vi "rio_veloster12.vi"() -> ()   [LabVIEW 2015]
uses:
  <vilib>/FPGAPlugInAG/cRIO-9113/niLvFpga_Open_cRIO-9113.vi
  <vilib>/rvi/interface/common/dynamic/niFpgaDynamicAddResources.vi
  <vilib>/FPGAPlugInAG/Dynamic/niLvFpga_Abort_Dynamic.vi
  <vilib>/FPGAPlugInAG/Dynamic/niLvFpga_Run_Dynamic.vi
  rio_Global.vi
  <vilib>/Utility/error.llb/Error Cluster From Error Code.vi
  <vilib>/rvi/errors/niLvFpgaAdjustHostInterfaceError.vi
  <vilib>/Instr/_visa.llb/VISA Configure Serial Port (Instr).vi
  <vilib>/Analysis/Matrix/Numeric/Conversions/Array To Matrix - RA2.vi
  <vilib>/Analysis/Matrix/Numeric/Multiply/Multiply - RM,RM.vi
  <vilib>/Analysis/Matrix/Numeric/Add/Add - RM,RM.vi
  <vilib>/Analysis/baseanly.llb/Real Inverse Matrix.vi
  <vilib>/Analysis/Matrix/Numeric/Subtract/Subtract - RM,RM.vi
  <vilib>/Analysis/Matrix/Numeric/Conversions/Array To Matrix - RA.vi
  <vilib>/Analysis/Matrix/Numeric/Multiply/Multiply - R,RM.vi
  <vilib>/Analysis/Matrix/Numeric/Conversions/Matrix To Array - RM.vi
  <vilib>/rvi/interface/nirviOpenFPGA/nirviOpenFPGA.xnode
  FPGA Bitfiles/autonomous_FPGATarget2_fpga4_FZHAM7r+pqE.lvbitx
  fpga/fpga4.vi
  <vilib>/rvi/interface/nirviMethod/nirviMethod.xnode
  <vilib>/rvi/interface/nirviReadWriteControl/nirviReadWriteControl.xnode
  <vilib>/Analysis/Matrix/NI_Matrix.lvlib
  <vilib>/Analysis/NI_AALBase.lvlib
  NiFpgaLv.dll
  <vilib>/rvi/interface/Simulation/niFpgaSimulationCallBeginRW.vi
panel:
  out "C_yaw_rate":dbl
  out "Time old":u32[](array[numeric])
  out "Heading":dbl
  out "H_GPS":dbl
  out "pos":dbl[](array[numeric])
  in  "GPS init":bool=TRUE
  out "pos_gps":dbl[](array[numeric]) format="%#_19f"
  out "dt":dbl
  out "Pos_time 10":i32
  out "FPGA":refnum<k20>
  in  "steer limit":dbl=100.0
  in  "buzz":bool
  out "hcount":u64=1
  out "hbias":dbl
  out "vcount":u64=1
  out "vgain":dbl=1.0
  out "T PWM":u16
  out "B PWM":u16
  out "mobileye":u8[](array[numeric])
  out "timer":u32
  out "Mobileye_time 100":u32
  out "pos error":dbl
  in  "Gear Manual":i32(slide)=1 scale=-1.0..1.0
  out "map":i32=2
  out "P, R, D":i32
  out "heading error":dbl
  out "POS init":bool
  out "VS_CAN":dbl
  in  "brake":bool
  in  "Slide":dbl(slide) min=-50.0 max=50.0 step=50.0 scale=-50.0..50.0
  out "Con_time 10":i32
  out "CAN_time 10":u32
  out "ecef ref":dbl[](array[numeric])
  out "h_gps":dbl
  out "get heading":bool
  out "get position":bool
  out "rt":dbl
  out "CAN Comm Enabled":bool
  in  "SPAS Enable":bool=TRUE
  in  "file write":bool
  out "data write":refnum<file>
  out "file rw error":errorcluster
  in  "Steer input":bool=TRUE
  in  "Manual Steering angle":dbl(knob) scale=-550.0..550.0
  out "Ref vel":dbl=1.0
  in  "Manual Speed":dbl
  in  "Velocity input":bool
  out "Auto":bool
  out "Run":bool
  out "E - STOP":bool
  # "P"
  # "R"
  # "D"
  # "Manual Steering angle"
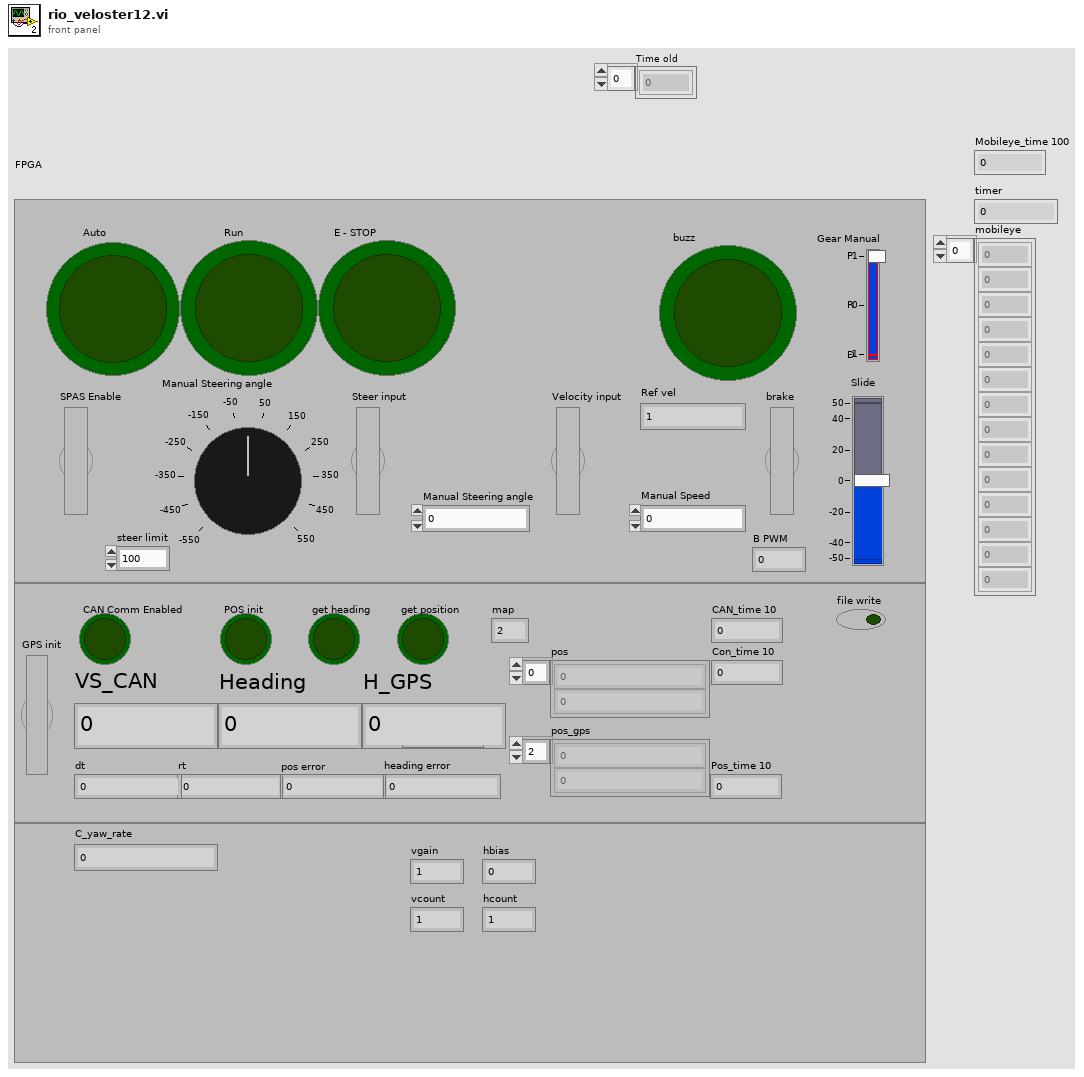
[diagram p1: front panel]
types:
  T1 = enum16{"open", "replace", "create", "open or create", "replace or create", "replace or create with confirmation"}
  T2 = cluster{"timestamp high":u32, "timestamp low":u32, "identifier":u32, "type":enum8{"Data Frame", "Remote Frame", "(reserved)", "(reserved) ", "(reserved)  ", "(reserved)   ", "Bus Error", "Transceiver Fault"}, "info A":u8, "info B":u8, "data length":u8, "data":u8[]}
  T3 = cluster{"identifier":u32, "timestamp":timestamp, "payload":u8[]}
  T4 = cluster{"connection ID":refnum<k16>, "net address":u32, "port":u16}
  T5 = cluster{"hash":i64, "sys time":i64, "mobileye":u8[]}
  T6 = cluster{"hash":i64, "sys time":i64, "time":dbl, "yaw_rate":dbl, "mdps torque":dbl, "mdps str_ang":dbl, "VS_CAN":dbl, "lat_accel":dbl, "mcp":dbl, "accel pedal value":dbl, "tps":dbl, "odometer":dbl, "battery voltage":dbl, "WHL_SPD_RR":dbl, "WHL_SPD_RL":dbl, "WHL_SPD_FR":dbl, "WHL_SPD_FL":dbl}
  T7 = cluster{"hash":i64, "sys time":i64, "ref_vel":dbl, "ref_steer":dbl, "alert":u8}
  T8 = cluster{"hash":i64, "sys time":i64, "ref_vel":dbl, "ref_steer":dbl}
  T9 = cluster{"hash":i64, "sys time":i64, "Auto":bool, "Run":bool, "Solenoid":bool, "T lim":bool, "brk_enc":u8, "B PWM":u16, "T PWM":u16, "ref_vel":dbl, "ref_bkr_enc":dbl, "ref_apv":dbl, "ref_steer":dbl}
  T10 = cluster{"hash":i64, "sys time":i64, "time":dbl, "x":dbl, "y":dbl, "h":dbl, "numSV":i32, "postype":i32, "lag":i32, "hordev":dbl, "lat":dbl, "lon":dbl, "hgt":dbl, "map_idx":i32}
  T11 = cluster{"output[0]":dbl, "output[1]":dbl, "output[2]":dbl, "output[3]":dbl, "output[4]":dbl, "output[5]":dbl, "output[6]":dbl, "output[7]":dbl, "output[8]":dbl, "output[9]":dbl, "output[10]":dbl, "output[11]":dbl, "output[12]":dbl, "output[13]":dbl, "output[14]":dbl}
  T12 = cluster{"hash":i64, "sys time":i64, "time":dbl, "speed":dbl, "heading":dbl, "lat":dbl, "lon":dbl}
  T13 = cluster{"output[0]":dbl, "output[1]":dbl, "output[2]":dbl, "output[3]":dbl, "output[4]":dbl, "output[5]":dbl, "output[6]":dbl}
  T14 = typedef "NI_Matrix.lvlib/RealMatrix.ctl" = dbl[][]
  T15 = cluster{"hash":i64, "sys time":i64, "dt":dbl, "x":dbl, "y":dbl, "speed":dbl, "heading":dbl, "yaw_rate":dbl}
  T16 = cluster{"Real 2D Array[0]":dbl, "Real 2D Array[1]":dbl, "Real 2D Array[2]":dbl, "Real 2D Array[3]":dbl, "Real 2D Array[4]":dbl}
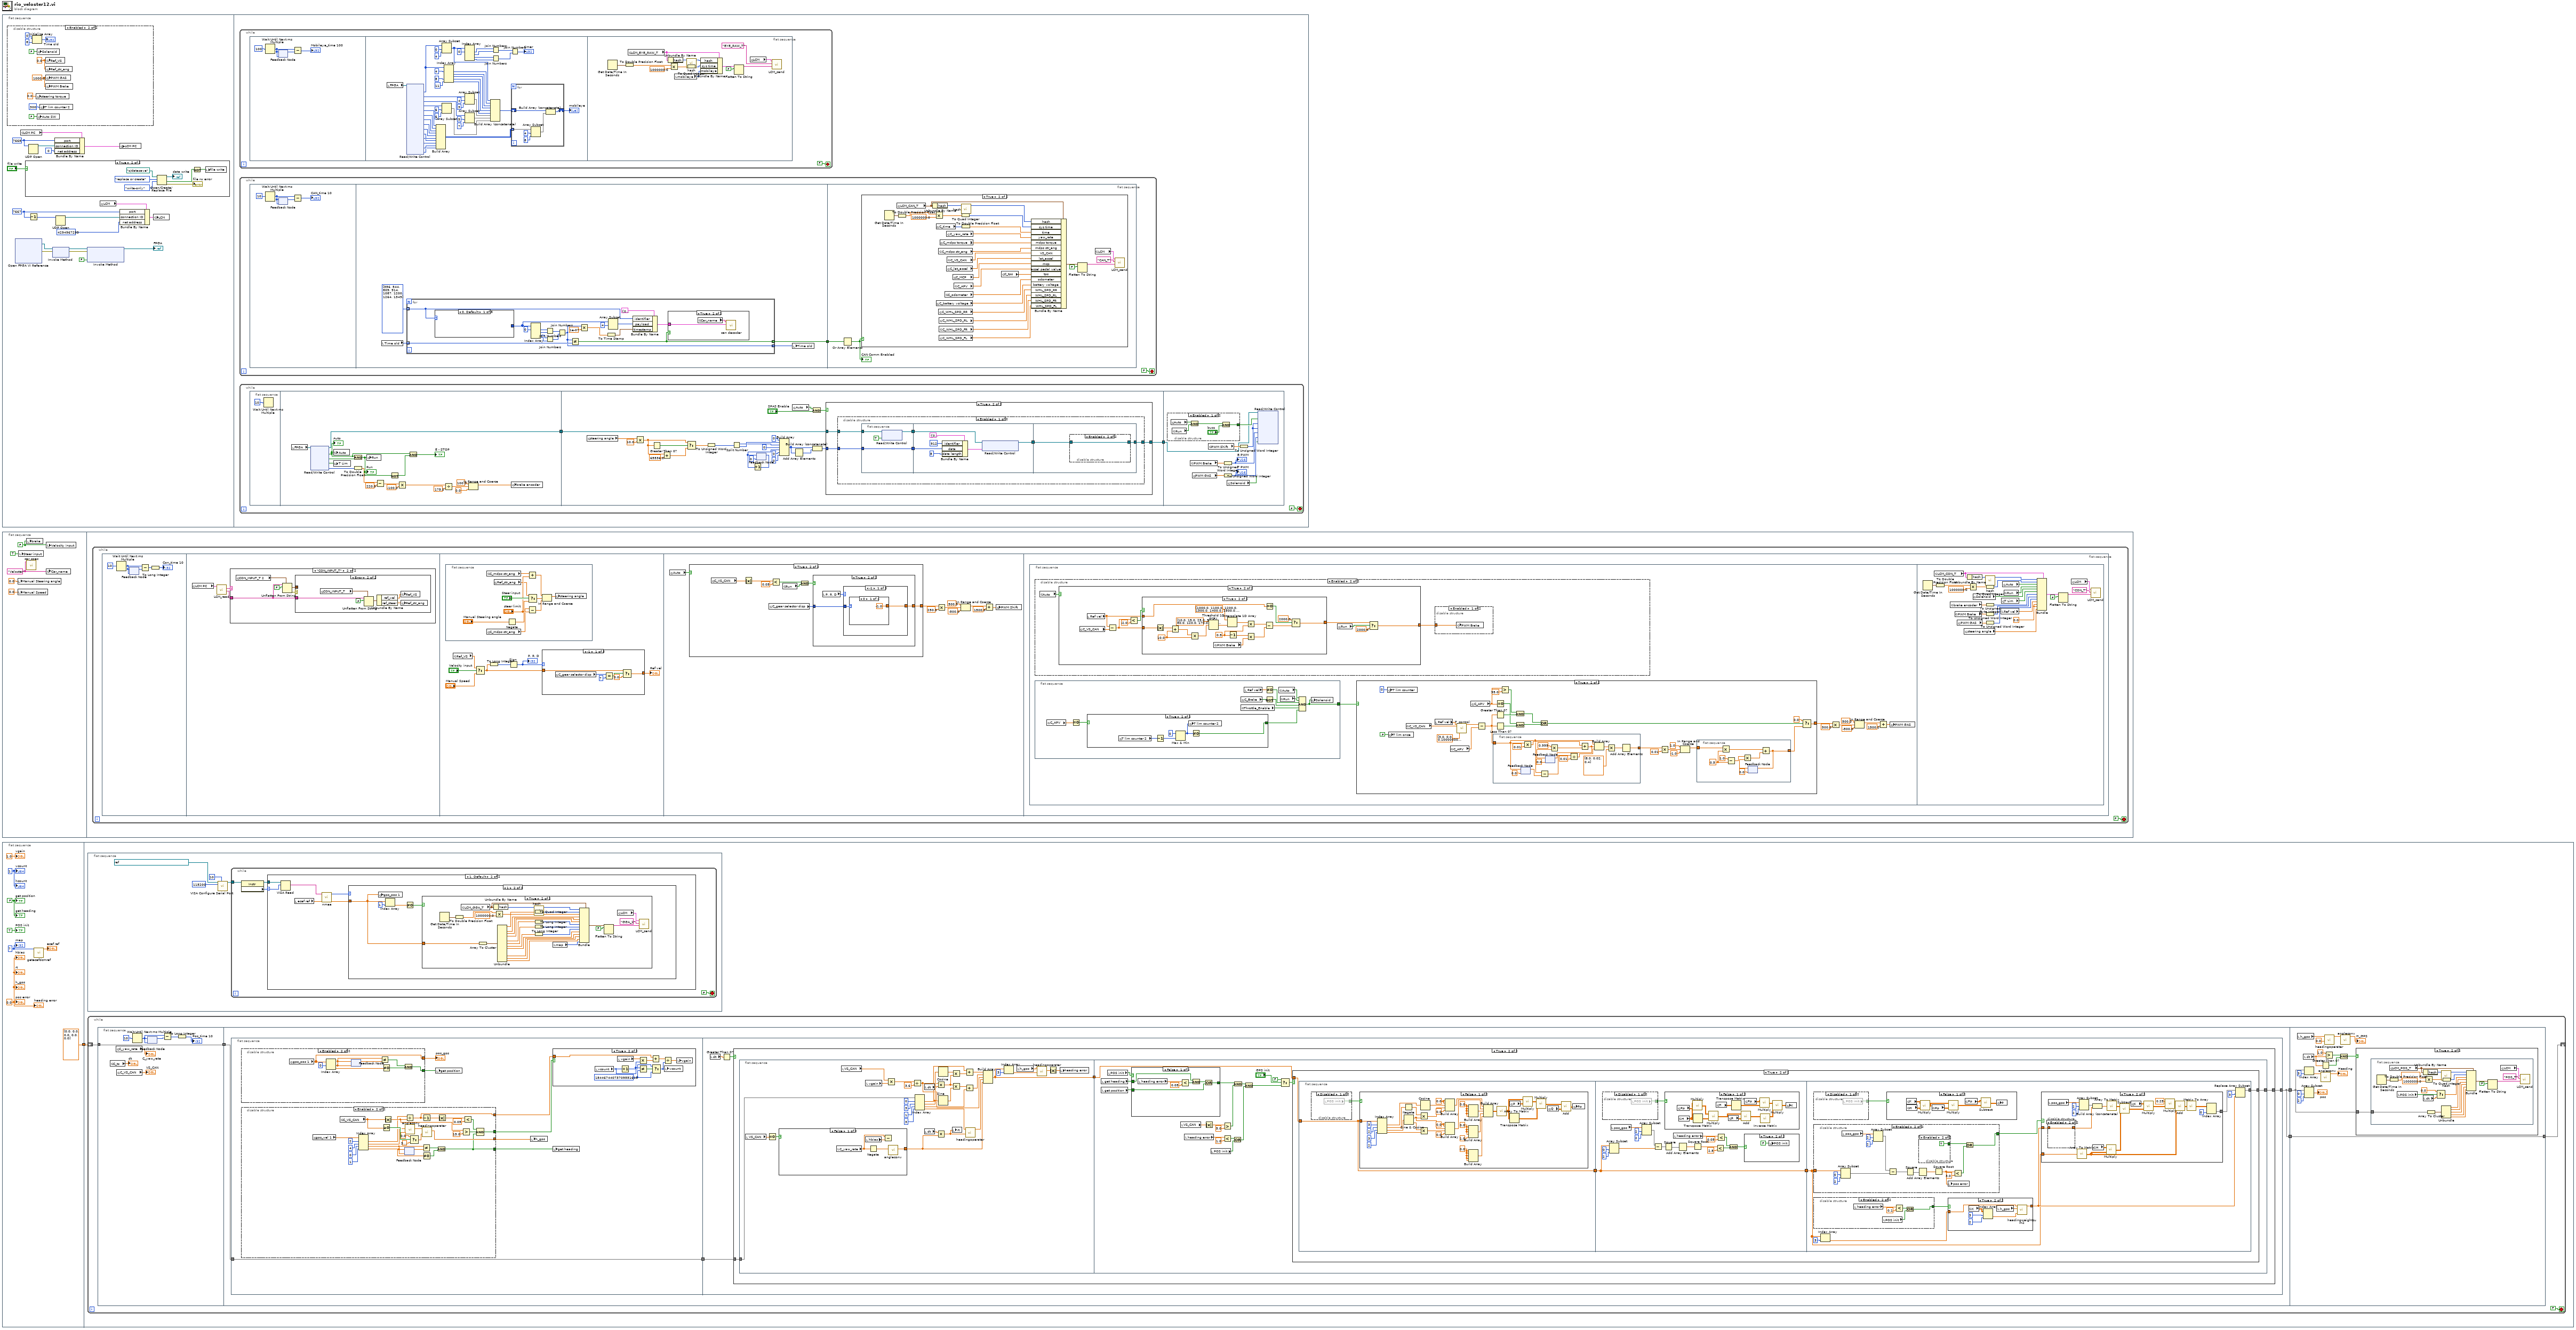
[diagram p0: block diagram]
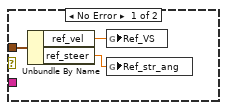
[diagram p3: hidden frame]
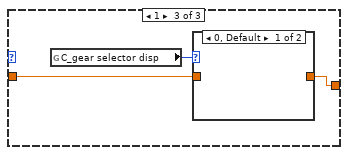
[diagram p5: hidden frame]
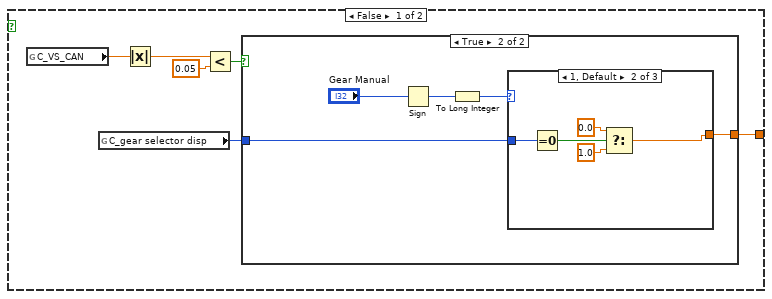
[diagram p7: hidden frame]
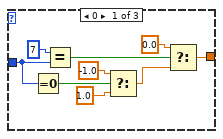
[diagram p9: hidden frame]
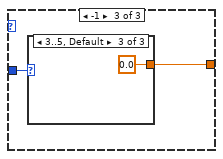
[diagram p10: hidden frame]
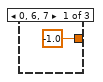
[diagram p11: hidden frame]
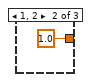
[diagram p12: hidden frame]
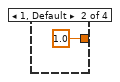
[diagram p14: hidden frame]
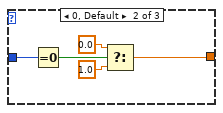
[diagram p17: hidden frame]
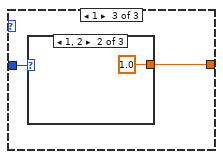
[diagram p18: hidden frame]
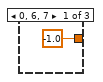
[diagram p19: hidden frame]
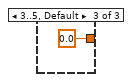
[diagram p20: hidden frame]
diagram:
  n1 = flat-sequence {
    frame #0 {
      w7 = u16 7668 ("port")
      w11 = u16 7667 ("port")
      n2 = disable-structure shown="Enabled" {
        frame Disabled {
        }
        frame Enabled {
          w24 = 0.0 ("Ref_str_ang")
          w25 = 1000.0 ("PWM GAS")
          n3 = Initialize Array(u32 0, 8 ("dimension size")) -> (→"Time old":u32[])
          n4 = global write "rio_Global.vi" "steering torque"(0.0 ("steering")) -> ()
          n5 = global write "rio_Global.vi" "Solenoid"(FALSE ("CAN A 1")) -> ()
          n6 = global write "rio_Global.vi" "Auto SW"(FALSE ("Auto SW")) -> ()
          n7 = global write "rio_Global.vi" "T lim counter 2"(u16 300 ("T lim counter 2")) -> ()
          n8 = global write "rio_Global.vi" "Ref_VS"(w24) -> ()
          n9 = global write "rio_Global.vi" "Ref_str_ang"(w24) -> ()
          n10 = global write "rio_Global.vi" "PWM GAS"(w25) -> ()
          n11 = global write "rio_Global.vi" "PWM Brake"(w25) -> ()
        }
      }
      n12 = xnode "Open FPGA VI Reference"() -> ("FPGA VI Reference Out"=w19:refnum<k20>, "error out"=w18:errorcluster)  [unwired: 2 in]
      n13 = global read "rio_Global.vi" "LCM PC"() -> (w3:T4)
      n14 = case shown="True" "file write" {
        frame False {
        }
        frame True {
          n15 = Open/Create/Replace File(file path (use dialog)=path "c:/datasave", operation (0:open)=T1."replace or create", access (0:read/write)=enum16{"read/write", "read-only", "write-only"}."write-only") -> (refnum out=→"data write":refnum<file>, cancelled=w32:bool, error out=→"file rw error":errorcluster)  [unwired: 3 in]
          n16 = Not(x=w32) -> (.not. x?=w31:bool)
          n17 = local write "file write"(w31) -> ()
        }
      }
      n18 = UDP Open(11:w7) -> (port=w9:refnum<k16>)  [unwired: 4 in, 2 out]
      n19 = Decrement(x=w11) -> (x-1=w10:u16)
      n20 = xnode "Invoke Method"("FPGA VI Reference In"=w19, "error in"=w18) -> ("FPGA VI Reference Out"=w17:refnum<k20>, "error out"=w16:errorcluster)
      n21 = Bundle By Name(cluster=w3, "port"=w7, "connection ID"=w9, "net address"=u32 0) -> (w4:T4)
      n22 = UDP Open(11:w10) -> (port=w13:refnum<k16>)  [unwired: 4 in, 2 out]
      n23 = xnode "Invoke Method"("FPGA VI Reference In"=w17, "error in"=w16, "Wait Until Done (F)"=FALSE) -> ("FPGA VI Reference Out"=→"FPGA":refnum<k20>)  [unwired: 1 out]
      n24 = global read "rio_Global.vi" "LCM"() -> (w6:T4)
      n25 = global write "rio_Global.vi" "LCM PC"(w4) -> ()
      n26 = Bundle By Name(cluster=w6, "port"=w11, "connection ID"=w13, "net address"=u32 4294967295) -> (w5:T4)
      n27 = global write "rio_Global.vi" "LCM"(w5) -> ()
    }
    frame #1 {
      n28 = while {
        stop <- FALSE stop-if-true
        n29 = flat-sequence {
          frame #0 {
            n30 = Wait Until Next ms Multiple(millisecond multiple=u32 100) -> (millisecond timer value=w132:u32)
            n31 = feedback #1(w132) -> (w130:u32)
            n32 = feedback-in #1(w132) -> ()
            n33 = Subtract(x=w132, y=w130) -> (x-y=→"Mobileye_time 100":u32)
          }
          frame #1 {
            n34 = local read "FPGA"() -> (w178:refnum<k20>)
            n35 = xnode "Read/Write Control"("FPGA VI Reference In"=w178) -> ("m 700"=w138:u8[], "m 760"=w174:u8[], "m 710"=w163:u8[], "m 711"=w159:u8[], "m 720"=w157:u8[], "m 721"=w156:u8[], "m 722"=w155:u8[], "m 723"=w154:u8[], "m 724"=w153:u8[], "m 725"=w152:u8[], "m 726"=w151:u8[], "m 727"=w150:u8[], "m 728"=w149:u8[], "m 729"=w148:u8[])  [unwired: 1 in, 2 out]
            n36 = Build Array(w157, w156, w155, w154, w153, w152, w151, w150, w149, w148) -> (w147:u8[][])
            n37 = Array Subset(array=w138, index=0, length=4) -> (w135:u8[])
            n38 = Array Subset(array=w159, index=6, length=6) -> (w158:u8[])
            n39 = Index Array(array=w138, index #1=4 ("index"), index #4=8 ("index"), index #5=11 ("index")) -> (element #1=w171:u8, element #2=w170:u8, element #3=w169:u8, element #4=w168:u8, element #5=w167:u8)  [unwired: 2 in]
            n40 = Index Array(array=w135, index #1=0 ("index")) -> (element #1=w144:u8, element #2=w143:u8, element #3=w142:u8, element #4=w141:u8)  [unwired: 3 in]
            n41 = Array Subset(array=w174, index=4, length=3) -> (w166:u8[])
            n42 = Array Subset(array=w163, index=5, length=7) -> (w162:u8[])
            n43 = Build Array (concatenate)(w135, w171, w170, w169, w168, w167, w166, w162, w158) -> (w146:u8[])
            n44 = Join Numbers(hi=w144, lo=w143) -> ((hi.lo)=w140:u16)
            n45 = Join Numbers(hi=w142, lo=w141) -> ((hi.lo)=w139:u16)
            n46 = Join Numbers(hi=w140, lo=w139) -> ((hi.lo)=→"timer":u32)
            n47 = for {
              tunnel: w147 -> [w180] mode=indexing
              shift-right: [w183] -> w133
              shift-left: w146 -> [w184]
              n48 = Array Subset(array=w180, index=4, length=8) -> (w179:u8[])
              n49 = Build Array (concatenate)(w184, w179) -> (w183:u8[])
            }
            "mobileye" <- w133
          }
          frame #2 {
            n50 = Get Date/Time In Seconds() -> (seconds since 1Jan1904=w191:timestamp)
            n51 = To Double Precision Float(number=w191) -> (double precision float=w190:dbl)
            n52 = global read "rio_Global.vi" "LCM_EYE_RAW_T"() -> (w185:T5)
            n53 = Unbundle By Name(w185) -> ("hash"=w198:i64)
            n54 = Multiply(x=w190, y=1000000.0) -> (x*y=w188:dbl)
            n55 = local read "mobileye"() -> (w192:u8[])
            n56 = call "hash.vi"("input"=w198) -> ("output"=w197:i64)  [unwired: 10 in]
            n57 = To Quad Integer(1:w188) -> (0:w187:i64)
            n58 = Bundle By Name(cluster=w185, "hash"=w197, "sys time"=w187, "mobileye"=w192) -> (w196:T5)
            n59 = Flatten To String(anything=w196, prepend array or string size? (T)=FALSE) -> (data string=w195:string)  [unwired: 2 in, 2 out]
            n60 = global read "rio_Global.vi" "LCM"() -> (w186:T4)
            n61 = call "LCM_send.vi"("DATA"=w195, "ID"="EYE_RAW_T", "LCM"=w186) -> ()  [unwired: 7 in, 2 out]
          }
        }
      }
      n62 = while {
        stop <- FALSE stop-if-true
        n63 = flat-sequence {
          tunnel: [w205] -> w199
          tunnel: w199 -> [w245]
          frame #0 {
            n64 = Wait Until Next ms Multiple(millisecond multiple=u32 10) -> (millisecond timer value=w203:u32)
            n65 = feedback #2(w203) -> (w202:u32)
            n66 = feedback-in #2(w203) -> ()
            n67 = Subtract(x=w203, y=w202) -> (x-y=→"CAN_time 10":u32)
          }
          frame #1 {
            n68 = local read "Time old"() -> (w207:u32[])
            n69 = for {
              tunnel: u32[] [356, 544, 809, 914, 1087, 1200, 1264, 1349] -> [w216] mode=indexing
              tunnel: w207 -> [w211] mode=indexing
              tunnel: [w210] -> w206 mode=indexing
              tunnel: [w209] -> w205 mode=indexing
              n70 = case shown="0, Default" w216 {
                tunnel: [_ w230 w232 w235 w236 w238 w240 w242] -> w215
                frame 0, Default {
                }
                frame 544 {
                  n71 = local read "FPGA"() -> (w231:refnum<k20>)
                  n72 = xnode "Read/Write Control"("FPGA VI Reference In"=w231) -> ("can 220"=w230:u8[])  [unwired: 1 in, 2 out]
                }
                frame 809 {
                  n73 = local read "FPGA"() -> (w233:refnum<k20>)
                  n74 = xnode "Read/Write Control"("FPGA VI Reference In"=w233) -> ("can 329"=w232:u8[])  [unwired: 1 in, 2 out]
                }
                frame 914 {
                  n75 = local read "FPGA"() -> (w234:refnum<k20>)
                  n76 = xnode "Read/Write Control"("FPGA VI Reference In"=w234) -> ("can 392"=w235:u8[])  [unwired: 1 in, 2 out]
                }
                frame 1087 {
                  n77 = local read "FPGA"() -> (w237:refnum<k20>)
                  n78 = xnode "Read/Write Control"("FPGA VI Reference In"=w237) -> ("can 43F"=w236:u8[])  [unwired: 1 in, 2 out]
                }
                frame 1200 {
                  n79 = local read "FPGA"() -> (w239:refnum<k20>)
                  n80 = xnode "Read/Write Control"("FPGA VI Reference In"=w239) -> ("can 4B0"=w238:u8[])  [unwired: 1 in, 2 out]
                }
                frame 1264 {
                  n81 = local read "FPGA"() -> (w241:refnum<k20>)
                  n82 = xnode "Read/Write Control"("FPGA VI Reference In"=w241) -> ("can 4F0"=w240:u8[])  [unwired: 1 in, 2 out]
                }
                frame 1349 {
                  n83 = local read "FPGA"() -> (w243:refnum<k20>)
                  n84 = xnode "Read/Write Control"("FPGA VI Reference In"=w243) -> ("can 545"=w242:u8[])  [unwired: 1 in, 2 out]
                }
              }
              n85 = Index Array(array=w215, index #1=0 ("index")) -> (element #1=w220:u8, element #2=w219:u8, element #3=w218:u8, element #4=w217:u8)  [unwired: 3 in]
              n86 = Join Numbers(hi=w220, lo=w219) -> ((hi.lo)=w223:u16)
              n87 = Join Numbers(hi=w218, lo=w217) -> ((hi.lo)=w224:u16)
              n88 = Join Numbers(hi=w223, lo=w224) -> ((hi.lo)=w210:u32)
              n89 = Not Equal?(x=w210, y=w211) -> (x != y?=w209:bool)
              n90 = Multiply(x=w210, y=1e-07) -> (x*y=w226:dbl)
              n91 = To Time Stamp(1:w226) -> (0:w227:timestamp)
              n92 = Array Subset(array=w215, index=4) -> (w213:u8[])  [unwired: 1 in]
              n93 = Bundle By Name(cluster=T3 {"identifier"=0, "timestamp"=timestamp(0 s since 1904-01-01), "payload"=[]} ("can cluster"), "identifier"=w216, "payload"=w213, "timestamp"=w227) -> (w212:T3)
              n94 = case shown="True" w209 {
                tunnel: w212 -> [_ w228]
                frame False {
                }
                frame True {
                  n95 = global read "rio_Global.vi" "Car_name"() -> (w229:string)
                  n96 = call "can decoder.vi"("can cluster"=w228, "name"=w229) -> ()  [unwired: 10 in]
                }
              }
            }
            n97 = local write "Time old"(w206) -> ()
          }
          frame #2 {
            n98 = Or Array Elements(Boolean array=w245) -> (logical OR=w244:bool)
            "CAN Comm Enabled" <- w244
            n99 = case shown="True" w244 {
              frame False {
              }
              frame True {
                n100 = Get Date/Time In Seconds() -> (seconds since 1Jan1904=w268:timestamp)
                n101 = global read "rio_Global.vi" "LCM_CAN_T"() -> (w248:T6)
                n102 = To Double Precision Float(number=w268) -> (double precision float=w267:dbl)
                n103 = Unbundle By Name(w248) -> ("hash"=w274:i64)
                n104 = Multiply(x=w267, y=1000000.0) -> (x*y=w265:dbl)
                n105 = global read "rio_Global.vi" "C_time"() -> (w263:u32)
                n106 = global read "rio_Global.vi" "C_battery voltage"() -> (w253:dbl)
                n107 = global read "rio_Global.vi" "C_mdps str_ang"() -> (w260:dbl)
                n108 = global read "rio_Global.vi" "C_WHL_SPD_RR"() -> (w252:dbl)
                n109 = global read "rio_Global.vi" "C_WHL_SPD_RL"() -> (w251:dbl)
                n110 = global read "rio_Global.vi" "C_WHL_SPD_FR"() -> (w250:dbl)
                n111 = global read "rio_Global.vi" "C_WHL_SPD_FL"() -> (w249:dbl)
                n112 = global read "rio_Global.vi" "C_mdps torque"() -> (w261:dbl)
                n113 = global read "rio_Global.vi" "C_odometer"() -> (w255:dbl)
                n114 = global read "rio_Global.vi" "C_yaw_rate"() -> (w262:dbl)
                n115 = global read "rio_Global.vi" "C_lat_accel"() -> (w258:dbl)
                n116 = global read "rio_Global.vi" "C_VS_CAN"() -> (w259:dbl)
                n117 = global read "rio_Global.vi" "C_MCP"() -> (w257:dbl)
                n118 = global read "rio_Global.vi" "C_APV"() -> (w256:dbl)
                n119 = To Quad Integer(1:w265) -> (0:w264:i64)
                n120 = call "hash.vi"("input"=w274) -> ("output"=w273:i64)  [unwired: 10 in]
                n121 = To Double Precision Float(number=w263) -> (double precision float=w272:dbl)
                n122 = global read "rio_Global.vi" "C_tps"() -> (w254:dbl)
                n123 = Bundle By Name(cluster=w248, "hash"=w273, "sys time"=w264, "time"=w272, "yaw_rate"=w262, "mdps torque"=w261, "mdps str_ang"=w260, "VS_CAN"=w259, "lat_accel"=w258, "mcp"=w257, "accel pedal value"=w256, "tps"=w254, "odometer"=w255, "battery voltage"=w253, "WHL_SPD_RR"=w252, "WHL_SPD_RL"=w251, "WHL_SPD_FR"=w250, "WHL_SPD_FL"=w249) -> (w271:T6)
                n124 = Flatten To String(anything=w271, prepend array or string size? (T)=FALSE) -> (data string=w270:string)  [unwired: 2 in, 2 out]
                n125 = global read "rio_Global.vi" "LCM"() -> (w246:T4)
                n126 = call "LCM_send.vi"("DATA"=w270, "ID"="CAN_T", "LCM"=w246) -> ()  [unwired: 7 in, 2 out]
              }
            }
          }
        }
      }
      n127 = while {
        stop <- FALSE stop-if-true
        n128 = flat-sequence {
          tunnel: [w43] -> w37
          tunnel: w37 -> [w60]
          tunnel: [w59] -> w36
          tunnel: w36 -> [w114]
          frame #0 {
            n129 = Wait Until Next ms Multiple(millisecond multiple=u32 10) -> ()  [unwired: 1 out]
          }
          frame #1 {
            n130 = local read "FPGA"() -> (w45:refnum<k20>)
            n131 = xnode "Read/Write Control"("FPGA VI Reference In"=w45) -> ("FPGA VI Reference Out"=w43:refnum<k20>, "Auto"=w44:bool, "Run"=w46:bool, "T Lim"=w40:bool, "brk enc"=w56:u8)  [unwired: 1 in, 1 out]
            "Auto" <- w44
            n132 = global write "rio_Global.vi" "Auto"(w44) -> ()
            n133 = global write "rio_Global.vi" "T Lim"(w40) -> ()
            n134 = And(x=w44, y=w46) -> (x .and. y?=w41:bool)
            "Run" <- w41
            n135 = To Double Precision Float(number=w56) -> (double precision float=w48:dbl)
            n136 = global write "rio_Global.vi" "Run"(w41) -> ()
            n137 = Subtract(x=w48, y=220.0) -> (x-y=w50:dbl)
            n138 = Not(x=w41) -> (.not. x?=w58:bool)
            n139 = Multiply(x=w50, y=-100.0) -> (x*y=w53:dbl)
            n140 = And(x=w44, y=w58) -> (x .and. y?=→"E - STOP":bool)
            n141 = Divide(x=w53, y=175.0) -> (x/y=w54:dbl)
            n142 = In Range and Coerce(upper limit=100.0, x=w54, lower limit=0.0) -> (coerced(x)=w42:dbl)  [unwired: 1 out]
            n143 = global write "rio_Global.vi" "brake encoder"(w42) -> ()
          }
          frame #2 {
            n144 = global read "rio_Global.vi" "steering angle"() -> (w83:dbl)
            n145 = Multiply(x=w83, y=10.0) -> (x*y=w65:dbl)
            n146 = Greater Than 0?(x=w65) -> (x > 0?=w64:bool)
            n147 = Add(x=w65, y=65536.0) -> (x+y=w67:dbl)
            n148 = Select(t=w65, s=w64, f=w67) -> (s? t:f=w68:dbl)
            n149 = To Unsigned Word Integer(number=w68) -> (unsigned 16bit integer=w69:u16)
            n150 = Split Number(x=w69) -> (hi(x)=w70:u8, lo(x)=w71:u8)
            n151 = feedback #3(u8 0 ("Con steer alivecnt")) -> (w80:u8)
            n152 = Increment(x=w80) -> (x+1=w79:u8)
            n153 = feedback-in #3(w79) -> ()
            n154 = Build Array(u8 0 ("Con steer status"), w71, w70, u8 0 ("element"), w80, u8 0 ("element"), u8 0 ("element")) -> (w76:u8[])
            n155 = global read "rio_Global.vi" "Auto"() -> (w82:bool)
            n156 = Add Array Elements(numeric array=w76) -> (sum=w75:u8)
            n157 = And(x=w82, y="SPAS Enable") -> (x .and. y?=w61:bool)
            n158 = Build Array (concatenate)(w76, w75) -> (w81:u8[])
            n159 = case shown="True" w61 {
              tunnel: w81 -> [_ w89]
              tunnel: w60 -> [w85 w88]
              tunnel: [w84 w87] -> w59
              frame False {
                n160 = xnode "Read/Write Control"("FPGA VI Reference In"=w85, "send can"=FALSE) -> ("FPGA VI Reference Out"=w84:refnum<k20>)  [unwired: 1 in, 1 out]
              }
              frame True {
                n161 = disable-structure shown="Enabled" {
                  disable-tunnel: w89 -> [w95 _]
                  disable-tunnel: w88 -> [w91 w113]
                  disable-tunnel: [w90 w113] -> w87
                  frame Enabled {
                    n162 = flat-sequence {
                      tunnel: w95 -> [w99]
                      tunnel: [w99] -> w94
                      tunnel: [w97] -> w93
                      tunnel: w91 -> [w96]
                      tunnel: w94 -> [w104]
                      tunnel: w93 -> [w102]
                      tunnel: [w101] -> w92
                      tunnel: w92 -> [w108]
                      tunnel: [w107] -> w90
                      frame #0 {
                        n163 = xnode "Read/Write Control"("FPGA VI Reference In"=w96, "send can"=TRUE) -> ("FPGA VI Reference Out"=w97:refnum<k20>)  [unwired: 1 in, 1 out]
                      }
                      frame #1 {
                        n164 = Bundle By Name(cluster=T2 {"timestamp high"=0, "timestamp low"=0, "identifier"=0, "type"=enum."Data Frame", "info A"=0, "info B"=0, "data length"=8, "data"=[0, 0, 0, 0, 0, 0, 0, 0]} ("Mod4/CAN1 input"), "identifier"=u32 912, "data"=w104, "data length"=u8 8) -> (w103:T2)
                        n165 = xnode "Read/Write Control"("FPGA VI Reference In"=w102, "Mod4/CAN1 input"=w103) -> ("FPGA VI Reference Out"=w101:refnum<k20>)  [unwired: 1 in, 1 out]
                      }
                      frame #2 {
                        n166 = disable-structure shown="Enabled" {
                          disable-tunnel: w108 -> [w111 w112]
                          disable-tunnel: [w109 w112] -> w107
                          frame Disabled {
                            n167 = xnode "Read/Write Control"("FPGA VI Reference In"=w111, "send can"=FALSE) -> ("FPGA VI Reference Out"=w109:refnum<k20>)  [unwired: 1 in, 1 out]
                          }
                          frame Enabled {
                          }
                        }
                      }
                    }
                  }
                  frame Disabled {
                  }
                }
              }
            }
          }
          frame #3 {
            n168 = disable-structure shown="Enabled" {
              disable-tunnel: [w125 _] -> w119
              frame Enabled {
                n169 = global read "rio_Global.vi" "Auto"() -> (w124:bool)
                n170 = global read "rio_Global.vi" "Run"() -> (w123:bool)
                n171 = Compound Arithmetic op=AND(w124, w123) -> (w127:bool)
                n172 = And(x=w127, y="buzz") -> (x .and. y?=w125:bool)
              }
              frame Disabled {
              }
            }
            n173 = global read "rio_Global.vi" "PWM Brake"() -> (w117:dbl)
            n174 = global read "rio_Global.vi" "PWM GAS"() -> (w116:dbl)
            n175 = global read "rio_Global.vi" "PWM Shift"() -> (w122:dbl)
            n176 = To Unsigned Word Integer(number=w117) -> (unsigned 16bit integer=w121:u16)
            "B PWM" <- w121
            n177 = To Unsigned Word Integer(number=w116) -> (unsigned 16bit integer=w118:u16)
            "T PWM" <- w118
            n178 = global read "rio_Global.vi" "Solenoid"() -> (w115:bool)
            n179 = To Unsigned Word Integer(number=w122) -> (unsigned 16bit integer=w120:u16)
            n180 = xnode "Read/Write Control"("FPGA VI Reference In"=w114, "Buzz"=w119, "S Pwm 1"=w120, "S Pwm 2"=w120, "B Pwm"=w121, "T Pwm"=w118, "Solenoid"=w115) -> ()  [unwired: 1 in, 2 out]
          }
        }
      }
    }
  }
  n181 = flat-sequence {
    frame #0 {
      w275 = "Veloster" ("Car_name")
      w279 = FALSE ("GPS init")
      n182 = local write "Manual Steering angle"(0.0 ("steer manual")) -> ()
      n183 = local write "Manual Speed"(0.0 ("Manual Speed")) -> ()
      n184 = local write "Steer input"(TRUE ("Steer input")) -> ()
      n185 = local write "brake"(w279) -> ()
      n186 = call "car_spec.vi"("Car_name"=w275) -> ()  [unwired: 5 in, 6 out]
      n187 = local write "Velocity input"(w279) -> ()
      n188 = global write "rio_Global.vi" "Car_name"(w275) -> ()
    }
    frame #1 {
      n189 = while {
        stop <- FALSE stop-if-true
        n190 = flat-sequence {
          frame #0 {
            n191 = Wait Until Next ms Multiple(millisecond multiple=u32 10) -> (millisecond timer value=w284:u32)
            n192 = feedback #4(w284) -> (w283:u32)
            n193 = feedback-in #4(w284) -> ()
            n194 = Subtract(x=w284, y=w283) -> (x-y=w282:u32)
            n195 = To Long Integer(number=w282) -> (32bit integer=→"Con_time 10":i32)
          }
          frame #1 {
            n196 = global read "rio_Global.vi" "LCM PC"() -> (w286:T4)
            n197 = call "LCM_read.vi"("LCM"=w286) -> ("data"=w288:string, "ID"=w287:string)  [unwired: 7 in, 2 out]
            n198 = case shown="\"CON_INPUT_T\"" w287 {
              tunnel: w288 -> [_ w289]
              frame "False", Default {
              }
              frame "CON_INPUT_T" {
                n199 = global read "rio_Global.vi" "CON_INPUT_T 2"() -> (w291:T7)
                n200 = Unflatten From String(type=w291, binary string=w289, data includes array or string size? (T)=FALSE) -> (value=w290:T7, error out=w292:errorcluster)  [unwired: 2 in, 1 out]
                n201 = case shown="Error" w292 {
                  tunnel: w290 -> [w296 _]
                  tunnel: w289 -> [_ w300]
                  frame No Error {
                    n202 = Unbundle By Name(w296) -> ("ref_vel"=w295:dbl, "ref_steer"=w294:dbl)
                    n203 = global write "rio_Global.vi" "Ref_VS"(w295) -> ()
                    n204 = global write "rio_Global.vi" "Ref_str_ang"(w294) -> ()
                  }
                  frame Error {
                    n205 = global read "rio_Global.vi" "CON_INPUT_T"() -> (w302:T8)
                    n206 = Unflatten From String(type=w302, binary string=w300, data includes array or string size? (T)=FALSE) -> (value=w297:T8)  [unwired: 2 in, 2 out]
                    n207 = Unbundle By Name(w297) -> ("ref_vel"=w299:dbl, "ref_steer"=w298:dbl)
                    n208 = global write "rio_Global.vi" "Ref_VS"(w299) -> ()
                    n209 = global write "rio_Global.vi" "Ref_str_ang"(w298) -> ()
                  }
                }
              }
            }
          }
          frame #2 {
            n210 = flat-sequence {
              frame #0 {
                n211 = global read "rio_Global.vi" "C_mdps str_ang"() -> (w323:dbl)
                n212 = global read "rio_Global.vi" "C_mdps str_ang"() -> (w322:dbl)
                n213 = global read "rio_Global.vi" "Ref_str_ang"() -> (w321:dbl)
                n214 = Negate(x="Manual Steering angle") -> (-x=w325:dbl)
                n215 = Add(x=w323, y="steer limit") -> (x+y=w329:dbl)
                n216 = Subtract(x=w322, y="steer limit") -> (x-y=w328:dbl)
                n217 = Select(t=w321, s="Steer input", f=w325) -> (s? t:f=w327:dbl)
                n218 = In Range and Coerce(upper limit=w329, x=w327, lower limit=w328) -> (coerced(x)=w320:dbl)  [unwired: 1 out]
                n219 = global write "rio_Global.vi" "steering angle"(w320) -> ()
              }
            }
            n220 = global read "rio_Global.vi" "Ref_VS"() -> (w303:dbl)
            n221 = Select(t=w303, s="Velocity input", f="Manual Speed") -> (s? t:f=w306:dbl)
            n222 = To Long Integer(number=w306) -> (32bit integer=w305:i32)
            n223 = Sign(1:w305) -> (0:w304:i32)
            "P, R, D" <- w304
            n224 = case shown="-1" w304 {
              tunnel: [w311 _ w318] -> w307
              tunnel: w306 -> [w313 _ w317]
              frame -1 {
                n225 = global read "rio_Global.vi" "C_gear selector disp"() -> (w310:u8)
                n226 = Equal?(x=w310, y=u8 7) -> (x = y?=w314:bool)
                n227 = Select(t=w313, s=w314, f=0.0) -> (s? t:f=w311:dbl)
              }
              frame 0, Default {
              }
              frame 1 {
                n228 = global read "rio_Global.vi" "C_gear selector disp"() -> (w316:u8)
                n229 = case shown="0, Default" w316 {
                  tunnel: [_ w319] -> w318
                  tunnel: w317 -> [_ w319]
                  frame 0, Default {
                  }
                  frame 4, 5 {
                  }
                }
              }
            }
            "Ref vel" <- w307
          }
          frame #3 {
            n230 = global read "rio_Global.vi" "Auto"() -> (w339:bool)
            n231 = case shown="True" w339 {
              tunnel: [w342 w377] -> w331
              frame False {
                n232 = global read "rio_Global.vi" "C_VS_CAN"() -> (w341:dbl)
                n233 = global read "rio_Global.vi" "C_gear selector disp"() -> (w340:u8)
                n234 = Absolute Value(x=w341) -> (abs(x)=w345:dbl)
                n235 = Less?(x=w345, y=0.05) -> (x < y?=w343:bool)
                n236 = case shown="True" w343 {
                  tunnel: [_ w349] -> w342
                  tunnel: w340 -> [_ w346]
                  frame False {
                  }
                  frame True {
                    n237 = Sign(1:"Gear Manual") -> (0:w350:i32)
                    n238 = To Long Integer(number=w350) -> (32bit integer=w348:i32)
                    n239 = case shown="1, Default" w348 {
                      tunnel: [w357 w362 w366] -> w349
                      tunnel: w346 -> [w351 w360 w365]
                      frame 0 {
                        n240 = Equal To 0?(x=w351) -> (x = 0?=w355:bool)
                        n241 = Equal?(x=u8 7 ("y"), y=w351) -> (x = y?=w359:bool)
                        n242 = Select(t=-1.0, s=w355, f=1.0) -> (s? t:f=w354:dbl)
                        n243 = Select(t=0.0, s=w359, f=w354) -> (s? t:f=w357:dbl)
                      }
                      frame 1, Default {
                        n244 = Equal To 0?(x=w360) -> (x = 0?=w364:bool)
                        n245 = Select(t=0.0, s=w364, f=1.0 ("t")) -> (s? t:f=w362:dbl)
                      }
                      frame -1 {
                        n246 = case shown="3..5, Default" w365 {
                          tunnel: [-1.0 1.0 0.0] -> w366
                          frame 0, 6, 7 {
                          }
                          frame 1, 2 {
                          }
                          frame 3..5, Default {
                          }
                        }
                      }
                    }
                  }
                }
              }
              frame True {
                n247 = global read "rio_Global.vi" "C_VS_CAN"() -> (w372:dbl)
                n248 = Absolute Value(x=w372) -> (abs(x)=w375:dbl)
                n249 = global read "rio_Global.vi" "C_gear selector disp"() -> (w370:u8)
                n250 = Less?(x=w375, y=0.05) -> (x < y?=w373:bool)
                n251 = global read "rio_Global.vi" "Run"() -> (w371:bool)
                n252 = And(x=w373, y=w371) -> (x .and. y?=w376:bool)
                n253 = case shown="True" w376 {
                  tunnel: [_ w380] -> w377
                  tunnel: w370 -> [_ w378]
                  frame False {
                  }
                  frame True {
                    n254 = local read "P, R, D"() -> (w379:i32)
                    n255 = case shown="-1" w379 {
                      tunnel: [w382 w387 w391] -> w380
                      tunnel: w378 -> [w381 w385 w390]
                      frame -1 {
                        n256 = case shown="0" w381 {
                          tunnel: [-1.0 ("t") 1.0 ("t") _ _] -> w382
                          frame 0 {
                          }
                          frame 1, Default {
                          }
                          frame 4, 8 {
                          }
                          frame 7 {
                          }
                        }
                      }
                      frame 0, Default {
                        n257 = Equal To 0?(x=w385) -> (x = 0?=w389:bool)
                        n258 = Select(t=0.0, s=w389, f=1.0 ("t")) -> (s? t:f=w387:dbl)
                      }
                      frame 1 {
                        n259 = case shown="1, 2" w390 {
                          tunnel: [-1.0 1.0 0.0] -> w391
                          frame 0, 6, 7 {
                          }
                          frame 1, 2 {
                          }
                          frame 3..5, Default {
                          }
                        }
                      }
                    }
                  }
                }
              }
            }
            n260 = Multiply(x=w331, y=250.0 ("S gain")) -> (x*y=w336:dbl)
            n261 = In Range and Coerce(upper limit=500.0, x=w336, lower limit=-500.0) -> (coerced(x)=w333:dbl)  [unwired: 1 out]
            n262 = Add(x=w333, y=1500.0) -> (x+y=w338:dbl)
            n263 = global write "rio_Global.vi" "PWM Shift"(w338) -> ()
          }
          frame #4 {
            n264 = flat-sequence {
              frame #0 {
                n265 = disable-structure shown="Enabled" {
                  frame Disabled {
                    n266 = global read "rio_Global.vi" "Auto"() -> (w404:bool)
                    n267 = case shown="True" w404 {
                      tunnel: [w445 w459] -> w405
                      frame False {
                        n268 = global read "rio_Global.vi" "C_MCP"() -> (w442:dbl)
                        n269 = global read "rio_Global.vi" "brake encoder"() -> (w438:dbl)
                        n270 = Multiply(x=w442, y=10.0) -> (x*y=w440:dbl)
                        n271 = Square Root(x=w440) -> (sqrt(x)=w439:dbl)
                        n272 = Not Equal To 0?(x=w438) -> (x != 0?=w444:bool)
                        n273 = Subtract(x=0.0, y=w439) -> (x-y=w446:dbl)
                        n274 = Select(t=w446, s=w444, f=0.0) -> (s? t:f=w445:dbl)
                      }
                      frame True {
                        n275 = global read "rio_Global.vi" "Run"() -> (w448:bool)
                        n276 = case shown="False" w448 {
                          tunnel: [w461 w466] -> w457
                          frame False {
                            n277 = global read "rio_Global.vi" "Const Brk FULL"() -> (w461:dbl)
                          }
                          frame True {
                            n278 = global read "rio_Global.vi" "C_VS_CAN"() -> (w462:dbl)
                            n279 = global read "rio_Global.vi" "Const Brk FULL"() -> (w465:dbl)
                            n280 = local read "Ref vel"() -> (w464:dbl)
                            n281 = Equal To 0?(x=w464) -> (x = 0?=w468:bool)
                            n282 = call "B_control.vi"("Ref vel"=w464, "VS_CAN"=w462) -> ("Ref Brk Enc"=w463:dbl)  [unwired: 17 in]
                            n283 = Select(t=w465, s=w468, f=w463) -> (s? t:f=w467:dbl)
                            n284 = Max & Min(x=w465, y=w467) -> (min(x,y)=w466:dbl)  [unwired: 1 out]
                          }
                        }
                        n285 = global read "rio_Global.vi" "C_MCP"() -> (w453:dbl)
                        n286 = global read "rio_Global.vi" "brake encoder"() -> (w449:dbl)
                        n287 = Multiply(x=w453, y=10.0) -> (x*y=w451:dbl)
                        n288 = Square Root(x=w451) -> (sqrt(x)=w450:dbl)
                        n289 = Subtract(x=w457, y=w450) -> (x-y=w458:dbl)
                        n290 = Equal To 0?(x=w449) -> (x = 0?=w455:bool)
                        n291 = Equal To 0?(x=w457) -> (x = 0?=w456:bool)
                        n292 = And(x=w455, y=w456) -> (x .and. y?=w454:bool)
                        n293 = Select(t=0.0, s=w454, f=w458) -> (s? t:f=w459:dbl)
                      }
                    }
                    n294 = flat-sequence {
                      tunnel: w405 -> [w433]
                      frame #0 {
                        w408 = 0.2 ("x")
                        n295 = Multiply(x=w433, y=-0.01) -> (x*y=w435:dbl)
                        n296 = In Range and Coerce(upper limit=1.0 ("x"), x=w435, lower limit=-1.0) -> (coerced(x)=w426:dbl)  [unwired: 1 out]
                        n297 = Subtract(x=1.0, y=w408) -> (x-y=w410:dbl)
                        n298 = Multiply(x=w426, y=w408) -> (x*y=w412:dbl)
                        n299 = feedback #5(0.0) -> (w409:dbl)
                        n300 = Multiply(x=w410, y=w409) -> (x*y=w411:dbl)
                        n301 = Add(x=w412, y=w411) -> (x+y=w427:dbl)
                        n302 = feedback-in #5(w427) -> ()
                        n303 = Multiply(x=w426, y=1.8 ("B P gain")) -> (x*y=w407:dbl)
                        n304 = call "deadzone.vi"("min"=-15.0, "max"=15.0, "x"=w427) -> ("dead zone"=w428:dbl)  [unwired: 8 in]
                        n305 = Multiply(x=w428, y=0.1 ("B D gain")) -> (x*y=w406:dbl)
                        n306 = Add(x=w407, y=w406) -> (x+y=w415:dbl)
                        n307 = Multiply(x=w415, y=600.0 ("B gain")) -> (x*y=w423:dbl)
                        n308 = Select(t=w423, s="brake", f="Slide") -> (s? t:f=w421:dbl)
                        n309 = In Range and Coerce(upper limit=500.0, x=w421, lower limit=-500.0) -> (coerced(x)=w420:dbl)  [unwired: 1 out]
                        n310 = Add(x=w420, y=1500.0) -> (x+y=w425:dbl)
                        n311 = global write "rio_Global.vi" "PWM Brake"(w425) -> ()
                      }
                    }
                  }
                  frame Enabled {
                    n312 = global read "rio_Global.vi" "Auto"() -> (w469:bool)
                    n313 = case shown="True" w469 {
                      tunnel: [1000.0 ("f") w473] -> w470
                      frame False {
                      }
                      frame True {
                        n314 = global read "rio_Global.vi" "C_VS_CAN"() -> (w480:dbl)
                        n315 = local read "Ref vel"() -> (w477:dbl)
                        n316 = Subtract(x=w477, y=w480) -> (x-y=w476:dbl)
                        n317 = Less?(x=w476, y=-2.0 ("lower limit")) -> (x < y?=w478:bool)
                        n318 = case shown="True" w478 {
                          tunnel: w476 -> [w481 w512]
                          tunnel: [w482 w502] -> w474
                          tunnel: w477 -> [w486 w503]
                          frame False {
                            n319 = Equal To 0?(x=w486) -> (x = 0?=w485:bool)
                            n320 = global read "rio_Global.vi" "PWM Brake"() -> (w494:dbl)
                            n321 = Greater?(x=w481, y=1.0) -> (0:w490:bool)
                            n322 = Multiply(x=w494, y=0.999) -> (x*y=w492:dbl)
                            n323 = Max & Min(x=w492, y=1000.0) -> (max(x,y)=w488:dbl)  [unwired: 1 out]
                            n324 = Select(t=1000.0, s=w490, f=w488) -> (s? t:f=w483:dbl)
                            n325 = Select(t=2000.0, s=w485, f=w483) -> (s? t:f=w482:dbl)
                          }
                          frame True {
                            w500 = 0.5 ("gain brake")
                            w509 = 10.0 ("y")
                            n326 = Absolute Value(x=w512) -> (abs(x)=w511:dbl)
                            n327 = Add(x=w511, y=w509) -> (x+y=w510:dbl)
                            n328 = Multiply(x=w510, y=w509) -> (x*y=w508:dbl)
                            n329 = Threshold 1D Array(2:w508, 3:dbl[] [10.0, 15.0, 25.0, 50.0, 80.0, 120.0, 170.0, 230.0, 290.0, 350.0, 420.0]) -> (0:w506:dbl)  [unwired: 1 in]
                            n330 = global read "rio_Global.vi" "PWM Brake"() -> (w498:dbl)
                            n331 = Interpolate 1D Array(1:w506, 2:dbl[] [1000.0, 1100.0, 1200.0, 1300.0, 1400.0, 1500.0, 1600.0, 1700.0, 1800.0, 1900.0, 2000.0]) -> (0:w501:dbl)
                            n332 = Decrement(x=w500) -> (x-1=w499:dbl)
                            n333 = Multiply(x=w501, y=w500) -> (x*y=w496:dbl)
                            n334 = Multiply(x=w499, y=w498) -> (x*y=w497:dbl)
                            n335 = Subtract(x=w496, y=w497) -> (x-y=w495:dbl)
                            n336 = Equal To 0?(x=w503) -> (x = 0?=w504:bool)
                            n337 = Select(t=2000.0, s=w504, f=w495) -> (s? t:f=w502:dbl)
                          }
                        }
                        n338 = global read "rio_Global.vi" "Run"() -> (w475:bool)
                        n339 = Select(t=w474, s=w475, f=2000.0) -> (s? t:f=w473:dbl)
                      }
                    }
                    n340 = disable-structure shown="Enabled" {
                      disable-tunnel: w470 -> [w514 _]
                      frame Enabled {
                        n341 = global write "rio_Global.vi" "PWM Brake"(w514) -> ()
                      }
                      frame Disabled {
                      }
                    }
                  }
                }
                n342 = flat-sequence {
                  tunnel: [w515] -> w395
                  frame #0 {
                    n343 = global read "rio_Global.vi" "C_APV"() -> (w520:dbl)
                    n344 = Equal To 0?(x=w520) -> (x = 0?=w522:bool)
                    n345 = case shown="True" w522 {
                      tunnel: [TRUE w530] -> w523
                      frame False {
                        n346 = global write "rio_Global.vi" "T lim counter 2"(u16 300 ("T lim counter 2")) -> ()
                      }
                      frame True {
                        n347 = global read "rio_Global.vi" "T lim counter 2"() -> (w528:u16)
                        n348 = Decrement(x=w528) -> (x-1=w531:u16)
                        n349 = Max & Min(x=u16 0, y=w531) -> (max(x,y)=w529:u16)  [unwired: 1 out]
                        n350 = global write "rio_Global.vi" "T lim counter 2"(w529) -> ()
                        n351 = Not Equal To 0?(x=w529) -> (x != 0?=w530:bool)
                      }
                    }
                    n352 = global read "rio_Global.vi" "Throttle_Enable"() -> (w516:bool)
                    n353 = global read "rio_Global.vi" "C_Brake"() -> (w517:bool)
                    n354 = local read "Ref vel"() -> (w521:dbl)
                    n355 = Not Equal To 0?(x=w521) -> (x != 0?=w525:bool)
                    n356 = Not(x=w517) -> (.not. x?=w524:bool)
                    n357 = global read "rio_Global.vi" "Auto"() -> (w519:bool)
                    n358 = global read "rio_Global.vi" "Run"() -> (w518:bool)
                    n359 = Compound Arithmetic op=AND(w519, w518, w525, w524, w516, w523) -> (w515:bool)
                    n360 = global write "rio_Global.vi" "Solenoid"(w515) -> ()
                  }
                }
                n361 = case shown="True" w395 {
                  tunnel: [w533 w576] -> w403
                  frame False {
                    n362 = flat-sequence {
                      tunnel: [w543] -> w533
                      frame #0 {
                        n363 = global read "rio_Global.vi" "T Lim"() -> (w534:bool)
                        n364 = case shown="True" w534 {
                          selector: w534 -> [_ w539]
                          frame False {
                            n365 = global write "rio_Global.vi" "T lim counter"(u16 0 ("T lim counter")) -> ()
                          }
                          frame True {
                            n366 = global write "rio_Global.vi" "T lim once"(w539) -> ()
                            n367 = global write "rio_Global.vi" "T lim counter 2"(u16 300 ("T lim counter 2")) -> ()
                            n368 = global read "rio_Global.vi" "T lim counter"() -> (w536:u16)
                            n369 = Increment(x=w536) -> (x+1=w541:u16)
                            n370 = Max & Min(x=u16 100, y=w541) -> (min(x,y)=w537:u16)  [unwired: 1 out]
                            n371 = global write "rio_Global.vi" "T lim counter"(w537) -> ()
                          }
                        }
                      }
                      frame #1 {
                        n372 = global read "rio_Global.vi" "T lim once"() -> (w542:bool)
                        n373 = case shown="True" w542 {
                          tunnel: [-1.0 ("t") w548] -> w543
                          frame False {
                          }
                          frame True {
                            n374 = global read "rio_Global.vi" "T lim counter"() -> (w545:u16)
                            n375 = Equal?(x=w545, y=u16 100) -> (x = y?=w547:bool)
                            n376 = Select(t=0.0, s=w547, f=-0.15) -> (s? t:f=w548:dbl)
                          }
                        }
                        n377 = global write "rio_Global.vi" "Throttle_Enable"(w542) -> ()
                      }
                    }
                  }
                  frame True {
                    n378 = global write "rio_Global.vi" "T lim counter"(u16 0 ("T lim counter")) -> ()
                    n379 = global write "rio_Global.vi" "T lim once"(FALSE ("T lim once")) -> ()
                    n380 = global read "rio_Global.vi" "C_VS_CAN"() -> (w556:dbl)
                    n381 = local read "Ref vel"() -> (w555:dbl)
                    n382 = global read "rio_Global.vi" "C_APV"() -> (w552:dbl)
                    n383 = call "T_control.vi"("Ref vel"=w555, "VS_CAN"=w556, "pid gain"=dbl[] [3.0, 0.0, 0.10000000000000003] ("pid gain 1")) -> ("Ref APS"=w553:dbl)  [unwired: 16 in]
                    n384 = global read "rio_Global.vi" "C_APV"() -> (w551:dbl)
                    n385 = Subtract(x=w553, y=w552) -> (x-y=w564:dbl)
                    n386 = flat-sequence {
                      tunnel: w564 -> [w597]
                      tunnel: [w594] -> w571
                      frame #0 {
                        n387 = feedback #6(0.0) -> (w602:dbl)
                        n388 = feedback-in #6(w597) -> ()
                        n389 = Multiply(x=w597, y=0.01) -> (x*y=w598:dbl)
                        n390 = Subtract(x=w597, y=w602) -> (x-y=w601:dbl)
                        n391 = feedback #7(0.0) -> (w593:dbl)
                        n392 = Multiply(x=0.999, y=w593) -> (x*y=w592:dbl)
                        n393 = Divide(x=w601, y=0.01) -> (x/y=w588:dbl)
                        n394 = Add(x=w598, y=w592) -> (x+y=w589:dbl)
                        n395 = feedback-in #7(w589) -> ()
                        n396 = Build Array(w597, w589, w588) -> (w596:dbl[])
                        n397 = Multiply(x=w596, y=dbl[] [8.0, 0.02, 0.4] ("pid gain 2")) -> (x*y=w595:dbl[])
                        n398 = Add Array Elements(numeric array=w595) -> (sum=w594:dbl)
                      }
                    }
                    n399 = Equal To 0?(x=w551) -> (x = 0?=w557:bool)
                    n400 = Greater Than 0?(x=w564) -> (x > 0?=w565:bool)
                    n401 = Less Than 0?(x=w564) -> (x < 0?=w558:bool)
                    n402 = Greater?(x=w551, y=95.0) -> (0:w566:bool)
                    n403 = And(x=w566, y=w565) -> (x .and. y?=w562:bool)
                    n404 = And(x=w557, y=w558) -> (x .and. y?=w563:bool)
                    n405 = Or(x=w562, y=w563) -> (x .or. y?=w561:bool)
                    n406 = Multiply(x=w571, y=0.01) -> (x*y=w569:dbl)
                    n407 = In Range and Coerce(upper limit=1.0 ("x"), x=w569, lower limit=-1.0) -> (coerced(x)=w560:dbl)  [unwired: 1 out]
                    n408 = flat-sequence {
                      tunnel: w560 -> [w578]
                      tunnel: [w584] -> w559
                      frame #0 {
                        w577 = 0.5 ("x")
                        n409 = Multiply(x=w578, y=w577) -> (x*y=w582:dbl)
                        n410 = Subtract(x=1.0, y=w577) -> (x-y=w580:dbl)
                        n411 = feedback #8(0.0) -> (w579:dbl)
                        n412 = Multiply(x=w580, y=w579) -> (x*y=w581:dbl)
                        n413 = Add(x=w582, y=w581) -> (x+y=w584:dbl)
                        n414 = feedback-in #8(w584) -> ()
                      }
                    }
                    n415 = Select(t=0.0 ("f"), s=w561, f=w559) -> (s? t:f=w576:dbl)
                  }
                }
                n416 = Multiply(x=w403, y=500.0 ("T gain")) -> (x*y=w401:dbl)
                n417 = In Range and Coerce(upper limit=500.0, x=w401, lower limit=-500.0) -> (coerced(x)=w397:dbl)  [unwired: 1 out]
                n418 = Add(x=w397, y=1500.0) -> (x+y=w396:dbl)
                n419 = global write "rio_Global.vi" "PWM GAS"(w396) -> ()
              }
              frame #1 {
                w607 = 0.0 ("ref_bkr_enc")
                n420 = Get Date/Time In Seconds() -> (seconds since 1Jan1904=w621:timestamp)
                n421 = global read "rio_Global.vi" "LCM_CON_T"() -> (w606:T9)
                n422 = To Double Precision Float(number=w621) -> (double precision float=w620:dbl)
                n423 = global read "rio_Global.vi" "brake encoder"() -> (w604:dbl)
                n424 = global read "rio_Global.vi" "PWM Brake"() -> (w611:dbl)
                n425 = global read "rio_Global.vi" "PWM GAS"() -> (w609:dbl)
                n426 = global read "rio_Global.vi" "steering angle"() -> (w616:dbl)
                n427 = Unbundle By Name(w606) -> ("hash"=w627:i64)
                n428 = Multiply(x=w620, y=1000000.0) -> (x*y=w618:dbl)
                n429 = global read "rio_Global.vi" "Solenoid"() -> (w615:bool)
                n430 = call "hash.vi"("input"=w627) -> ("output"=w626:i64)  [unwired: 10 in]
                n431 = To Quad Integer(1:w618) -> (0:w617:i64)
                n432 = To Unsigned Byte Integer(number=w604) -> (unsigned 8bit integer=w603:u8)
                n433 = To Unsigned Word Integer(number=w611) -> (unsigned 16bit integer=w610:u16)
                n434 = To Unsigned Word Integer(number=w609) -> (unsigned 16bit integer=w608:u16)
                n435 = local read "Ref vel"() -> (w622:dbl)
                n436 = global read "rio_Global.vi" "T Lim"() -> (w612:bool)
                n437 = global read "rio_Global.vi" "Auto"() -> (w614:bool)
                n438 = global read "rio_Global.vi" "Run"() -> (w613:bool)
                n439 = Bundle(cluster=w606, "hash"=w626, "sys time"=w617, "Auto"=w614, "Run"=w613, "Solenoid"=w615, "T lim"=w612, "brk_enc"=w603, "B PWM"=w610, "T PWM"=w608, "ref_vel"=w622, "ref_bkr_enc"=w607, "ref_apv"=w607, "ref_steer"=w616) -> (w623:T9)
                n440 = Flatten To String(anything=w623, prepend array or string size? (T)=FALSE) -> (data string=w624:string)  [unwired: 2 in, 2 out]
                n441 = global read "rio_Global.vi" "LCM"() -> (w605:T4)
                n442 = call "LCM_send.vi"("DATA"=w624, "ID"="CON_T", "LCM"=w605) -> ()  [unwired: 7 in, 2 out]
              }
            }
          }
        }
      }
    }
  }
  n443 = flat-sequence {
    tunnel: [dbl[] [0.0, 0.0, 0.0, 0.0, 0.0] ("pos(i)")] -> w1
    tunnel: w1 -> [w637]
    frame #0 {
      w633 = 7 ("map")
      w630 = FALSE ("get heading")
      w636 = u64 1
      w635 = 0.0 ("dh_hat")
      n444 = call "getecefdcmref.vi"("map name"=w633) -> ("XYZ"=→"ecef ref":dbl[])  [unwired: 10 in, 4 out]
      "vgain" <- 1.0 ("initH")
      "vcount" <- w636
      "hbias" <- w635
      "hcount" <- w636
      "get heading" <- w630
      "get position" <- w630
      "heading error" <- w635
      "h_gps" <- w635
      "rt" <- w635
      "pos error" <- w635
      "map" <- w633
      "POS init" <- TRUE ("pos linit")
    }
    frame #1 {
      n445 = flat-sequence {
        frame #0 {
          n446 = call-poly "VISA Configure Serial Port"("VISA resource name"=refnum<visa-resource-name> "USB0::0x1546::0x01A6::NI-VISA-0::1::RAW", "timeout (10sec)"=u32 10, "baud rate (9600)"=u32 115200) -> ("VISA resource name out"=w641:refnum<visa-resource-name>)  [unwired: 11 in, 1 out]
          n447 = while {
            tunnel: w641 -> [w645]
            stop <- FALSE stop-if-true
            n448 = property class="Instr"(reference=w645) -> (reference out=w644:refnum<visa-resource-name>, "Serial Settings:Number of Bytes at Serial Port"=w642:u32)  [unwired: 1 in, 1 out]
            n449 = case shown="1, Default" w642 {
              selector: w642 -> [_ w647]
              tunnel: w644 -> [_ w651]
              frame 0 {
                n450 = Wait (ms)(milliseconds to wait=u32 10) -> ()  [unwired: 1 out]
              }
              frame 1, Default {
                n451 = VISA Read(VISA resource name=w651, byte count=w647) -> (read buffer=w652:string)  [unwired: 1 in, 3 out]
                n452 = local read "ecef ref"() -> (w648:dbl[])
                n453 = call "nmea.vi"("ecef ref"=w648, "NMEA"=w652) -> ("output"=w650:dbl[], "type"=w649:u32)  [unwired: 8 in]
                n454 = case shown="1" w649 {
                  tunnel: w650 -> [_ w654 w687]
                  frame 0, Default {
                  }
                  frame 1 {
                    n455 = global write "rio_Global.vi" "gps_pos 1"(w654) -> ()
                    n456 = Index Array(array=w654, index=1) -> (element=w656:dbl)
                    n457 = Not Equal To 0?(x=w656) -> (x != 0?=w653:bool)
                    n458 = case shown="True" w653 {
                      tunnel: w654 -> [_ w676]
                      frame False {
                      }
                      frame True {
                        n459 = Get Date/Time In Seconds() -> (seconds since 1Jan1904=w661:timestamp)
                        n460 = To Double Precision Float(number=w661) -> (double precision float=w660:dbl)
                        n461 = global read "rio_Global.vi" "LCM_GGA_T"() -> (w685:T10)
                        n462 = Array To Cluster(array=w676) -> (cluster=w684:T11)
                        n463 = Unbundle By Name(w685) -> ("hash"=w681:i64)
                        n464 = Multiply(x=w660, y=1000000.0) -> (x*y=w658:dbl)
                        n465 = Unbundle(w684) -> ("output[0]"=w686:dbl, "output[2]"=w675:dbl, "output[3]"=w674:dbl, "output[4]"=w673:dbl, "output[6]"=w672:dbl, "output[7]"=w670:dbl, "output[8]"=w668:dbl, "output[9]"=w666:dbl, "output[12]"=w665:dbl, "output[13]"=w664:dbl, "output[14]"=w663:dbl)  [unwired: 4 out]
                        n466 = call "hash.vi"("input"=w681) -> ("output"=w680:i64)  [unwired: 10 in]
                        n467 = To Quad Integer(1:w658) -> (0:w657:i64)
                        n468 = To Long Integer(number=w672) -> (32bit integer=w671:i32)
                        n469 = To Long Integer(number=w670) -> (32bit integer=w669:i32)
                        n470 = To Long Integer(number=w668) -> (32bit integer=w667:i32)
                        n471 = local read "map"() -> (w662:i32)
                        n472 = Bundle(cluster=w685, "hash"=w680, "sys time"=w657, "time"=w686, "x"=w675, "y"=w674, "h"=w673, "numSV"=w671, "postype"=w669, "lag"=w667, "hordev"=w666, "lat"=w665, "lon"=w664, "hgt"=w663, "map_idx"=w662) -> (w682:T10)
                        n473 = Flatten To String(anything=w682, prepend array or string size? (T)=FALSE) -> (data string=w678:string)  [unwired: 2 in, 2 out]
                        n474 = global read "rio_Global.vi" "LCM"() -> (w677:T4)
                        n475 = call "LCM_send.vi"("DATA"=w678, "ID"="GGA_1", "LCM"=w677) -> ()  [unwired: 7 in, 2 out]
                      }
                    }
                  }
                  frame 2 {
                    n476 = flat-sequence {
                      tunnel: w687 -> [w689]
                      frame #0 {
                        n477 = Index Array(array=w689, index=1) -> (element=w691:dbl)
                        n478 = Not Equal To 0?(x=w691) -> (x != 0?=w688:bool)
                        n479 = case shown="True" w688 {
                          tunnel: w689 -> [_ w710]
                          frame False {
                          }
                          frame True {
                            n480 = Get Date/Time In Seconds() -> (seconds since 1Jan1904=w696:timestamp)
                            n481 = To Double Precision Float(number=w696) -> (double precision float=w695:dbl)
                            n482 = global read "rio_Global.vi" "LCM_RMC_T"() -> (w711:T12)
                            n483 = Unbundle By Name(w711) -> ("hash"=w707:i64)
                            n484 = Multiply(x=w695, y=1000000.0) -> (x*y=w693:dbl)
                            n485 = Array To Cluster(array=w710) -> (cluster=w709:T13)
                            n486 = To Quad Integer(1:w693) -> (0:w692:i64)
                            n487 = call "hash.vi"("input"=w707) -> ("output"=w706:i64)  [unwired: 10 in]
                            n488 = Unbundle(w709) -> ("output[0]"=w701:dbl, "output[2]"=w700:dbl, "output[4]"=w699:dbl, "output[5]"=w698:dbl, "output[6]"=w697:dbl)  [unwired: 2 out]
                            n489 = Bundle(cluster=w711, "hash"=w706, "sys time"=w692, "time"=w701, "speed"=w700, "heading"=w699, "lat"=w698, "lon"=w697) -> (w702:T12)
                            n490 = Flatten To String(anything=w702, prepend array or string size? (T)=FALSE) -> (data string=w704:string)  [unwired: 2 in, 2 out]
                            n491 = global read "rio_Global.vi" "LCM"() -> (w703:T4)
                            n492 = call "LCM_send.vi"("DATA"=w704, "ID"="RMC_1", "LCM"=w703) -> ()  [unwired: 7 in, 2 out]
                          }
                        }
                      }
                    }
                    n493 = global write "rio_Global.vi" "gps_vel 1"(w687) -> ()
                  }
                }
              }
            }
          }
        }
      }
      n494 = while {
        shift-right: [w712] -> _
        shift-left: w637 -> [w713]
        stop <- FALSE stop-if-true
        n495 = flat-sequence {
          tunnel: [w726] -> w716
          tunnel: w713 -> [w726]
          tunnel: w716 -> [w729]
          tunnel: [w728] -> w715
          tunnel: [w728] -> w714
          tunnel: [w1147] -> w712
          tunnel: w715 -> [w1148]
          tunnel: w714 -> [w1147]
          frame #0 {
            n496 = global read "rio_Global.vi" "C_ts"() -> (→"dt":dbl)
            n497 = global read "rio_Global.vi" "C_yaw_rate"() -> (→"C_yaw_rate":dbl)
            n498 = global read "rio_Global.vi" "C_VS_CAN"() -> (→"VS_CAN":dbl)
            n499 = Wait Until Next ms Multiple(millisecond multiple=u32 10) -> (millisecond timer value=w724:u32)
            n500 = feedback #9(w724) -> (w723:u32)
            n501 = feedback-in #9(w724) -> ()
            n502 = Subtract(x=w724, y=w723) -> (x-y=w722:u32)
            n503 = To Long Integer(number=w722) -> (32bit integer=→"Pos_time 10":i32)
          }
          frame #1 {
            n504 = flat-sequence {
              tunnel: w729 -> [w736]
              tunnel: [w736] -> w727
              tunnel: [w858] -> w728
              tunnel: w727 -> [w859]
              frame #0 {
                n505 = disable-structure shown="Enabled" {
                  disable-tunnel: [w756 w757] -> w731
                  disable-tunnel: [w737 w758] -> w730
                  frame Disabled {
                    n506 = global read "rio_Global.vi" "gps_pos 1"() -> (w753:dbl[])
                    n507 = global read "rio_Global.vi" "gps_pos 2"() -> (w740:dbl[])
                    n508 = Add(x=w753, y=w740) -> (x+y=w755:dbl[])
                    n509 = Index Array(array=w753, index #1=0 ("index")) -> (element #1=w752:dbl, element #2=w751:dbl)  [unwired: 1 in]
                    n510 = Index Array(array=w740, index #1=0 ("index")) -> (element #1=w741:dbl, element #2=w742:dbl)  [unwired: 1 in]
                    n511 = feedback #10(w752) -> (w750:dbl)
                    n512 = feedback-in #10(w752) -> ()
                    n513 = feedback #11(w741) -> (w743:dbl)
                    n514 = feedback-in #11(w741) -> ()
                    n515 = Not Equal?(x=w752, y=w750) -> (x != y?=w749:bool)
                    n516 = Not Equal?(x=w741, y=w743) -> (x != y?=w744:bool)
                    n517 = Not Equal To 0?(x=w751) -> (x != 0?=w748:bool)
                    n518 = Not Equal To 0?(x=w742) -> (x != 0?=w745:bool)
                    n519 = And(x=w749, y=w748) -> (x .and. y?=w738:bool)
                    n520 = And(x=w744, y=w745) -> (x .and. y?=w739:bool)
                    n521 = And(x=w738, y=w739) -> (x .and. y?=w756:bool)
                    n522 = Multiply(x=w755, y=0.5) -> (x*y=w737:dbl[])
                  }
                  frame Enabled {
                    n523 = global read "rio_Global.vi" "gps_pos 1"() -> (w758:dbl[])
                    n524 = Index Array(array=w758, index #1=0 ("index")) -> (element #1=w764:dbl, element #2=w763:dbl)  [unwired: 1 in]
                    n525 = feedback #12(w764) -> (w762:dbl)
                    n526 = feedback-in #12(w764) -> ()
                    n527 = Not Equal?(x=w764, y=w762) -> (x != y?=w761:bool)
                    n528 = Not Equal To 0?(x=w763) -> (x != 0?=w760:bool)
                    n529 = And(x=w761, y=w760) -> (x .and. y?=w757:bool)
                  }
                }
                "pos_gps" <- w730
                n530 = disable-structure shown="Enabled" {
                  disable-tunnel: [w811 w841] -> w735
                  disable-tunnel: [w810 w822] -> w734
                  disable-tunnel: [w782 w833] -> w733
                  disable-tunnel: [w770 w829] -> w732
                  frame Disabled {
                    n531 = global read "rio_Global.vi" "gps_vel 1"() -> (w809:dbl[])
                    n532 = global read "rio_Global.vi" "gps_vel 2"() -> (w788:dbl[])
                    n533 = Index Array(array=w809, index #1=0 ("index"), index #2=1 ("index"), index #3=4 ("index"), index #4=2 ("index")) -> (element #1=w800:dbl, element #2=w805:dbl, element #3=w802:dbl, element #4=w774:dbl)
                    n534 = Index Array(array=w788, index #1=0 ("index"), index #2=1 ("index"), index #3=4 ("index"), index #4=2 ("index")) -> (element #1=w797:dbl, element #2=w792:dbl, element #3=w795:dbl, element #4=w773:dbl)
                    n535 = local read "VS_CAN"() -> (w766:dbl)
                    n536 = local read "VS_CAN"() -> (w765:dbl)
                    n537 = Add(x=w774, y=w773) -> (x+y=w772:dbl)
                    n538 = call "angleconv.vi"("deg"=w802) -> ("rad"=w785:dbl)  [unwired: 9 in, 1 out]
                    n539 = call "angleconv.vi"("deg"=w795) -> ("rad"=w784:dbl)  [unwired: 9 in, 1 out]
                    n540 = Not Equal To 0?(x=w792) -> (x != 0?=w793:bool)
                    n541 = feedback #13(0.0 ("Real Matrix Element")) -> (w799:dbl)
                    n542 = feedback-in #13(w800) -> ()
                    n543 = feedback #14(0.0 ("Real Matrix Element")) -> (w798:dbl)
                    n544 = feedback-in #14(w797) -> ()
                    n545 = Not Equal?(x=w800, y=w799) -> (x != y?=w806:bool)
                    n546 = Not Equal?(x=w797, y=w798) -> (x != y?=w791:bool)
                    n547 = Greater Or Equal To 0?(x=w765) -> (x >= 0?=w814:bool)
                    n548 = Not Equal To 0?(x=w805) -> (x != 0?=w804:bool)
                    n549 = Absolute Value(x=w766) -> (abs(x)=w767:dbl)
                    n550 = Multiply(x=w772, y=0.5) -> (x*y=w781:dbl)
                    n551 = call "headingweightsum.vi"("a"=0.5, "h1"=w784, "h2"=w785) -> ("a*h2+(1-a)*h1"=w813:dbl)  [unwired: 8 in]
                    n552 = And(x=w806, y=w804) -> (x .and. y?=w787:bool)
                    n553 = And(x=w791, y=w793) -> (x .and. y?=w786:bool)
                    n554 = Divide(x=w781, y=w767) -> (x/y=w782:dbl)
                    n555 = Select(t=0.0, s=w814, f=3.141592653589793) -> (s? t:f=w812:dbl)
                    n556 = Decrement(x=w782) -> (x-1=w778:dbl)
                    n557 = call "headingoperater.vi"("h1"=w812, "h2"=w813) -> ("h2-h1"=w811:dbl)  [unwired: 8 in, 1 out]
                    n558 = And(x=w787, y=w786) -> (x .and. y?=w810:bool)
                    n559 = Absolute Value(x=w778) -> (abs(x)=w779:dbl)
                    n560 = Greater?(x=w767, y=15.0) -> (0:w768:bool)
                    n561 = Less?(x=w779, y=0.05) -> (x < y?=w771:bool)
                    n562 = Compound Arithmetic op=AND(w768, w771, w810) -> (w770:bool)
                  }
                  frame Enabled {
                    n563 = global read "rio_Global.vi" "gps_vel 1"() -> (w840:dbl[])
                    n564 = global read "rio_Global.vi" "C_VS_CAN"() -> (w817:dbl)
                    n565 = Index Array(array=w840, index #1=2 ("index"), index #2=4 ("index"), index #3=0 ("index"), index #4=1 ("index")) -> (element #1=w820:dbl, element #2=w818:dbl, element #3=w825:dbl, element #4=w836:dbl)
                    n566 = Greater Or Equal To 0?(x=w817) -> (x >= 0?=w843:bool)
                    n567 = Absolute Value(x=w817) -> (abs(x)=w827:dbl)
                    n568 = feedback #15(w825) -> (w834:dbl)
                    n569 = feedback-in #15(w825) -> ()
                    n570 = Divide(x=w820, y=w827) -> (x/y=w833:dbl)
                    n571 = call "angleconv.vi"("deg"=w818) -> ("rad"=w826:dbl)  [unwired: 9 in, 1 out]
                    n572 = Select(t=0.0, s=w843, f=3.141592653589793) -> (s? t:f=w842:dbl)
                    n573 = Not Equal?(x=w825, y=w834) -> (x != y?=w837:bool)
                    n574 = Decrement(x=w833) -> (x-1=w830:dbl)
                    n575 = Not Equal To 0?(x=w836) -> (x != 0?=w835:bool)
                    n576 = call "headingoperater.vi"("h1"=w842, "h2"=w826) -> ("h2-h1"=w841:dbl)  [unwired: 8 in, 1 out]
                    n577 = And(x=w837, y=w835) -> (x .and. y?=w822:bool)
                    n578 = Absolute Value(x=w830) -> (abs(x)=w831:dbl)
                    n579 = Greater?(x=w827, y=15.0) -> (0:w823:bool)
                    n580 = Less?(x=w831, y=0.05) -> (x < y?=w824:bool)
                    n581 = Compound Arithmetic op=AND(w824, w823, w822) -> (w829:bool)
                  }
                }
                n582 = local write "get position"(w731) -> ()
                n583 = local write "h_gps"(w735) -> ()
                n584 = case shown="True" w732 {
                  tunnel: w733 -> [_ w853]
                  frame False {
                  }
                  frame True {
                    w847 = u64 18446744073709551615
                    n585 = local read "vcount"() -> (w850:u64)
                    n586 = local read "vgain"() -> (w855:dbl)
                    n587 = Increment(x=w850) -> (x+1=w849:u64)
                    n588 = Multiply(x=w855, y=w850) -> (x*y=w854:dbl)
                    n589 = Not Equal?(x=w850, y=w847) -> (x != y?=w848:bool)
                    n590 = Add(x=w853, y=w854) -> (x+y=w852:dbl)
                    n591 = Select(t=w849, s=w848, f=w847) -> (s? t:f=w846:u64)
                    n592 = Divide(x=w852, y=w846) -> (x/y=w851:dbl)
                    n593 = local write "vcount"(w846) -> ()
                    n594 = local write "vgain"(w851) -> ()
                  }
                }
                n595 = local write "get heading"(w734) -> ()
              }
              frame #1 {
                n596 = local read "dt"() -> (w857:dbl)
                n597 = Greater Than 0?(x=w857) -> (x > 0?=w856:bool)
                n598 = case shown="True" w856 {
                  tunnel: w859 -> [w860 w863]
                  tunnel: [w860 w862] -> w858
                  frame False {
                  }
                  frame True {
                    n599 = flat-sequence {
                      tunnel: w863 -> [w897]
                      tunnel: [w875] -> w861
                      tunnel: [w925] -> w862
                      tunnel: w861 -> [w924]
                      frame #0 {
                        n600 = local read "VS_CAN"() -> (w864:dbl)
                        n601 = Equal To 0?(x=w864) -> (x = 0?=w867:bool)
                        n602 = case shown="False" w867 {
                          tunnel: [w899 _] -> w866
                          frame False {
                            n603 = local read "C_yaw_rate"() -> (w898:dbl)
                            n604 = local read "hbias"() -> (w901:dbl)
                            n605 = Negate(x=w898) -> (-x=w900:dbl)
                            n606 = Subtract(x=w898, y=w901) -> ()  [unwired: 1 out]
                            n607 = call "angleconv.vi"("deg"=w900) -> ("rad"=w899:dbl)  [unwired: 9 in, 1 out]
                          }
                          frame True {
                            w905 = u64 18446744073709551615
                            n608 = local read "hcount"() -> (w908:u64)
                            n609 = local read "hbias"() -> (w911:dbl)
                            n610 = Increment(x=w908) -> (x+1=w907:u64)
                            n611 = local read "C_yaw_rate"() -> (w902:dbl)
                            n612 = Not Equal?(x=w908, y=w905) -> (x != y?=w906:bool)
                            n613 = Multiply(x=w911, y=w908) -> (x*y=w910:dbl)
                            n614 = Add(x=w902, y=w910) -> (x+y=w909:dbl)
                            n615 = Select(t=w907, s=w906, f=w905) -> (s? t:f=w904:u64)
                            n616 = local write "hcount"(w904) -> ()
                            n617 = Divide(x=w909, y=w904) -> (x/y=w903:dbl)
                            n618 = local write "hbias"(w903) -> ()
                          }
                        }
                        n619 = local read "VS_CAN"() -> (w865:dbl)
                        n620 = local read "vgain"() -> (w870:dbl)
                        n621 = Multiply(x=w865, y=w870) -> (x*y=w869:dbl)
                        n622 = Divide(x=w869, y=3.6) -> (x/y=w868:dbl)
                        n623 = Index Array(array=w897, index #1=0 ("index"), index #2=3 ("index"), index #3=1 ("index"), index #4=3 ("index")) -> (element #1=w891:dbl, element #2=w889:dbl, element #3=w885:dbl, element #4=w880:dbl)
                        n624 = local read "dt"() -> (w894:dbl)
                        n625 = local read "dt"() -> (w878:dbl)
                        n626 = Multiply(x=w868, y=w894) -> (x*y=w890:dbl)
                        n627 = Multiply(x=w878, y=w866) -> (x*y=w871:dbl)
                        n628 = Cosine(x=w889) -> (cos(x)=w895:dbl)
                        n629 = Sine(x=w889) -> (sin(x)=w888:dbl)
                        n630 = Multiply(x=w895, y=w890) -> (x*y=w892:dbl)
                        n631 = Multiply(x=w890, y=w888) -> (x*y=w887:dbl)
                        n632 = local write "rt"(w871) -> ()
                        n633 = Add(x=w891, y=w892) -> (x+y=w884:dbl)
                        n634 = Add(x=w887, y=w885) -> (x+y=w883:dbl)
                        n635 = call "headingoperater.vi"("h1"=w871, "h2"=w880) -> ("h2+h1"=w879:dbl)  [unwired: 8 in, 1 out]
                        n636 = Build Array(w884, w883, w868, w879, w866) -> (w875:dbl[])
                        n637 = Index Array(array=w875, index=3) -> (element=w874:dbl)
                        n638 = local read "h_gps"() -> (w873:dbl)
                        n639 = call "headingoperater.vi"("h1"=w874, "h2"=w873) -> ("h2-h1"=w877:dbl)  [unwired: 8 in, 1 out]
                        n640 = Absolute Value(x=w877) -> (abs(x)=w872:dbl)
                        n641 = local write "heading error"(w872) -> ()
                      }
                      frame #1 {
                        n642 = local read "get heading"() -> (w931:bool)
                        n643 = local read "get position"() -> (w930:bool)
                        n644 = local read "POS init"() -> (w917:bool)
                        n645 = case shown="False" w917 {
                          tunnel: w931 -> [w934 w941]
                          tunnel: w930 -> [w938 w940]
                          tunnel: [w932 w939] -> w927
                          frame False {
                            n646 = local read "heading error"() -> (w935:dbl)
                            n647 = Less?(x=w935, y=0.05) -> (x < y?=w936:bool)
                            n648 = And(x=w934, y=w936) -> (x .and. y?=w933:bool)
                            n649 = Or(x=w933, y=w938) -> (x .or. y?=w932:bool)
                          }
                          frame True {
                            n650 = disable-structure shown="Enabled" {
                              disable-tunnel: w941 -> [w944 w946]
                              disable-tunnel: w940 -> [w943 w945]
                              disable-tunnel: [w942 w947] -> w939
                              frame Disabled {
                                n651 = And(x=w944, y=w943) -> (x .and. y?=w942:bool)
                              }
                              frame Enabled {
                                n652 = Or(x=w946, y=w945) -> (x .or. y?=w947:bool)
                              }
                            }
                          }
                        }
                        n653 = local read "VS_CAN"() -> (w912:dbl)
                        n654 = local read "heading error"() -> (w920:dbl)
                        n655 = Absolute Value(x=w912) -> (abs(x)=w929:dbl)
                        n656 = local read "POS init"() -> (w918:bool)
                        n657 = Greater?(x=w929, y=5.0) -> (0:w926:bool)
                        n658 = Less?(x=w920, y=1.0) -> (x < y?=w919:bool)
                        n659 = Or(x=w919, y=w918) -> (x .or. y?=w921:bool)
                        n660 = And(x=w927, y=w926) -> (x .and. y?=w922:bool)
                        n661 = And(x=w922, y=w921) -> (x .and. y?=w915:bool)
                        n662 = Select(t=FALSE, s="GPS init", f=w915) -> (s? t:f=w914:bool)
                        n663 = case shown="True" w914 {
                          tunnel: [w952 w980] -> w925
                          tunnel: w924 -> [w953 w983]
                          frame False {
                            n664 = local read "VS_CAN"() -> (w948:dbl)
                            n665 = local read "POS init"() -> (w955:bool)
                            n666 = Equal To 0?(x=w948) -> (x = 0?=w954:bool)
                            n667 = local read "GPS init"() -> (w949:bool)
                            n668 = And(x=w955, y=w954) -> (x .and. y?=w951:bool)
                            n669 = Or(x=w951, y=w949) -> (x .or. y?=w950:bool)
                            n670 = case shown="True" w950 {
                              tunnel: w953 -> [w956 w957]
                              tunnel: [w956 w959] -> w952
                              tunnel: w949 -> [_ w958]
                              frame False {
                              }
                              frame True {
                                n671 = case shown="False" w958 {
                                tunnel: [w970 w979] -> w959
                                tunnel: w957 -> [w965 w973]
                                frame True {
                                n672 = Index Array(array=w965, index #1=2 ("index")) -> (element #2=w960:dbl, element #3=w963:dbl)  [unwired: 2 in, 1 out]
                                n673 = local write "GPS init"(FALSE ("GPS init")) -> ()
                                n674 = local read "pos_gps"() -> (w966:dbl[])
                                n675 = Index Array(array=w966, index #1=2 ("index")) -> (element #1=w968:dbl, element #2=w967:dbl)  [unwired: 1 in]
                                n676 = local read "h_gps"() -> (w961:dbl)
                                n677 = Build Array(w968, w967, w960, w961, w963) -> (w970:dbl[])
                                }
                                frame False {
                                w972 = 0.0 ("element")
                                n678 = Index Array(array=w973, index=3) -> (element=w971:dbl)
                                n679 = local read "pos_gps"() -> (w975:dbl[])
                                n680 = Index Array(array=w975, index #1=2 ("index")) -> (element #1=w977:dbl, element #2=w976:dbl)  [unwired: 1 in]
                                n681 = Build Array(w977, w976, w972, w971, w972) -> (w979:dbl[])
                                }
                                }
                              }
                            }
                          }
                          frame True {
                            n682 = flat-sequence {
                              tunnel: w983 -> [w985]
                              tunnel: [w985] -> w982
                              tunnel: w982 -> [w1029]
                              tunnel: [w1029] -> w981
                              tunnel: w981 -> [w1058]
                              tunnel: [w1062] -> w980
                              frame #0 {
                                n683 = disable-structure shown="Disabled" {
                                disable-tunnel: [w986 _] -> w984
                                frame Disabled {
                                n684 = local read "POS init"() -> (w986:bool)
                                }
                                frame Enabled {
                                }
                                }
                                n685 = case shown="False" w984 {
                                tunnel: w985 -> [w987 _]
                                frame False {
                                w996 = 0.0 ("element")
                                w1000 = 0.0 ("element")
                                w1002 = 0.0 ("element")
                                w1004 = 0.0 ("element")
                                w1006 = 0.0 ("element")
                                n686 = Index Array(array=w987, index #1=3 ("index"), index #2=2 ("index"), index #3=3 ("index"), index #4=2 ("index")) -> (element #1=w1016:dbl, element #2=w1018:dbl, element #3=w1021:dbl, element #4=w1010:dbl)
                                n687 = Negate(x=w1018) -> (-x=w1017:dbl)
                                n688 = Sine & Cosine(0:w1021) -> (1:w1013:dbl, 2:w1011:dbl)
                                n689 = Multiply(x=w1017, y=w1013) -> (x*y=w1014:dbl)
                                n690 = Multiply(x=w1011, y=w1010) -> (x*y=w1009:dbl)
                                n691 = Cosine(x=w1016) -> (cos(x)=w1015:dbl)
                                n692 = Build Array(w1006, w1006, w1015, w1014, 0.0 ("element")) -> (w1008:dbl[])
                                n693 = Build Array(w1004, w1004, w1013, w1009, 0.0 ("element")) -> (w1007:dbl[])
                                n694 = Build Array(w1002, w1002, w1002, w1002, w1002) -> (w1001:dbl[])
                                n695 = Build Array(w1000, w1000, w1000, w1000, 1.0 ("element")) -> (w998:dbl[])
                                n696 = Build Array(w996, w996, w996, w996, w996) -> (w997:dbl[])
                                n697 = Build Array(w1008, w1007, w1001, w998, w997) -> (w994:dbl[][])
                                n698 = call-poly <vilib>:"Array To Matrix.vi"("Real 2D Array"=w994) -> ("Real Matrix"=w992:T14)
                                n699 = global read "rio_Global.vi" "P"() -> (w995:T14)
                                n700 = Transpose Matrix(1:w992) -> (0:w991:T14)
                                n701 = call-poly <vilib>:"Multiply.vi"("Real Matrix B"=w995, "Real Matrix A"=w992) -> ("A * B"=w993:T14)
                                n702 = call-poly <vilib>:"Multiply.vi"("Real Matrix B"=w991, "Real Matrix A"=w993) -> ("A * B"=w990:T14)
                                n703 = global read "rio_Global.vi" "Q"() -> (w989:T14)
                                n704 = call-poly <vilib>:"Add.vi"("Real Matrix B"=w989, "Real Matrix A"=w990) -> ("A + B"=w988:T14)
                                n705 = global write "rio_Global.vi" "Pp"(w988) -> ()
                                }
                                frame True {
                                }
                                }
                              }
                              frame #1 {
                                n706 = disable-structure shown="Disabled" {
                                disable-tunnel: [w1042 _] -> w1023
                                frame Disabled {
                                n707 = local read "POS init"() -> (w1042:bool)
                                }
                                frame Enabled {
                                }
                                }
                                n708 = Array Subset(array=w1029, index=0, length=2) -> (w1036:dbl[])
                                n709 = local read "pos_gps"() -> (w1032:dbl[])
                                n710 = Array Subset(array=w1032, index=2, length=2) -> (w1035:dbl[])
                                n711 = Subtract(x=w1035, y=w1036) -> (x-y=w1037:dbl[])
                                n712 = Square(x=w1037) -> (x^2=w1038:dbl[])
                                n713 = case shown="False" w1023 {
                                frame False {
                                n714 = global read "rio_Global.vi" "Pp"() -> (w1055:T14)
                                n715 = global read "rio_Global.vi" "H"() -> (w1054:T14)
                                n716 = call-poly <vilib>:"Multiply.vi"("Real Matrix B"=w1055, "Real Matrix A"=w1054) -> ("A * B"=w1053:T14)
                                n717 = Transpose Matrix(1:w1054) -> (0:w1052:T14)
                                n718 = call-poly <vilib>:"Multiply.vi"("Real Matrix B"=w1052, "Real Matrix A"=w1053) -> ("A * B"=w1051:T14)
                                n719 = global read "rio_Global.vi" "H"() -> (w1049:T14)
                                n720 = global read "rio_Global.vi" "R"() -> (w1050:T14)
                                n721 = Transpose Matrix(1:w1049) -> (0:w1047:T14)
                                n722 = call-poly <vilib>:"Add.vi"("Real Matrix B"=w1050, "Real Matrix A"=w1051) -> ("A + B"=w1045:T14)
                                n723 = global read "rio_Global.vi" "Pp"() -> (w1048:T14)
                                n724 = call-poly <vilib>:"Multiply.vi"("Real Matrix B"=w1047, "Real Matrix A"=w1048) -> ("A * B"=w1046:T14)
                                n725 = call-poly <vilib>:"Inverse Matrix.vi"("Input Matrix"=w1045) -> ("Inverse Matrix"=w1044:T14)  [unwired: 1 in, 1 out]
                                n726 = call-poly <vilib>:"Multiply.vi"("Real Matrix B"=w1044, "Real Matrix A"=w1046) -> ("A * B"=w1043:T14)
                                n727 = global write "rio_Global.vi" "K"(w1043) -> ()
                                }
                                frame True {
                                }
                                }
                                n728 = local read "heading error"() -> (w1041:dbl)
                                n729 = Add Array Elements(numeric array=w1038) -> (sum=w1039:dbl)
                                n730 = Square Root(x=w1039) -> (sqrt(x)=w1028:dbl)
                                n731 = Less?(x=w1028, y=2.5) -> (x < y?=w1025:bool)
                                n732 = Less?(x=w1041, y=0.05) -> (x < y?=w1026:bool)
                                n733 = And(x=w1026, y=w1025) -> (x .and. y?=w1024:bool)
                                n734 = case shown="True" w1024 {
                                frame False {
                                }
                                frame True {
                                n735 = local write "POS init"(FALSE ("Kalman init")) -> ()
                                }
                                }
                              }
                              frame #2 {
                                n736 = disable-structure shown="Disabled" {
                                disable-tunnel: [w1067 _] -> w1057
                                frame Disabled {
                                n737 = local read "POS init"() -> (w1067:bool)
                                }
                                frame Enabled {
                                }
                                }
                                n738 = disable-structure shown="Enabled" {
                                disable-tunnel: [w1081 w1083] -> w1060
                                disable-tunnel: w1058 -> [_ w1092]
                                frame Disabled {
                                n739 = local read item#-1() -> (w1081)
                                }
                                frame Enabled {
                                n740 = Array Subset(array=w1092, index=0, length=2) -> (w1090:dbl[])
                                n741 = local read "pos_gps"() -> (w1095:dbl[])
                                n742 = Array Subset(array=w1095, index=2, length=2) -> (w1091:dbl[])
                                n743 = Subtract(x=w1091, y=w1090) -> (x-y=w1089:dbl[])
                                n744 = Square(x=w1089) -> (x^2=w1088:dbl[])
                                n745 = Add Array Elements(numeric array=w1088) -> (sum=w1087:dbl)
                                n746 = disable-structure shown="Enabled" {
                                disable-tunnel: [w1098 TRUE ("Kalman init")] -> w1085
                                frame Disabled {
                                n747 = local read item#-1() -> (w1098)
                                }
                                frame Enabled {
                                }
                                }
                                n748 = Square Root(x=w1087) -> (sqrt(x)=w1082:dbl)
                                n749 = local write "pos error"(w1082) -> ()
                                n750 = Less?(x=w1082, y=3.0) -> (x < y?=w1084:bool)
                                n751 = Or(x=w1085, y=w1084) -> (x .or. y?=w1083:bool)
                                }
                                }
                                n752 = disable-structure shown="Enabled" {
                                disable-tunnel: [w1075 w1076] -> w1061
                                frame Disabled {
                                n753 = local read item#-1() -> (w1075)
                                }
                                frame Enabled {
                                n754 = local read "heading error"() -> (w1079:dbl)
                                n755 = local read "POS init"() -> (w1077:bool)
                                n756 = Less?(x=w1079, y=0.1) -> (x < y?=w1078:bool)
                                n757 = Or(x=w1078, y=w1077) -> (x .or. y?=w1076:bool)
                                }
                                }
                                n758 = Index Array(array=w1058, index=3) -> (element=w1065:dbl)
                                n759 = case shown="False" w1057 {
                                frame False {
                                n760 = global read "rio_Global.vi" "K"() -> (w1074:T14)
                                n761 = global read "rio_Global.vi" "H"() -> (w1073:T14)
                                n762 = call-poly <vilib>:"Multiply.vi"("Real Matrix B"=w1073, "Real Matrix A"=w1074) -> ("A * B"=w1072:T14)
                                n763 = global read "rio_Global.vi" "Pp"() -> (w1071:T14)
                                n764 = call-poly <vilib>:"Multiply.vi"("Real Matrix B"=w1071, "Real Matrix A"=w1072) -> ("A * B"=w1070:T14)
                                n765 = global read "rio_Global.vi" "Pp"() -> (w1069:T14)
                                n766 = call-poly <vilib>:"Subtract.vi"("Real Matrix B"=w1070, "Real Matrix A"=w1069) -> ("A - B"=w1068:T14)
                                n767 = global write "rio_Global.vi" "P"(w1068) -> ()
                                }
                                frame True {
                                }
                                }
                                n768 = case shown="True" w1061 {
                                tunnel: w1065 -> [w1124 w1131]
                                tunnel: [w1124 w1126] -> w1059
                                frame False {
                                }
                                frame True {
                                n769 = global read "rio_Global.vi" "K"() -> (w1130:T14)
                                n770 = Index Array(array=w1130, index (row)=3, index (col)=2 ("disabled index (col)")) -> (element=w1127:dbl)
                                n771 = local read "h_gps"() -> (w1125:dbl)
                                n772 = call "headingweightsum2.vi"("a"=w1127, "h2"=w1125, "h1"=w1131) -> ("a*h2+(1-a)*h1"=w1126:dbl)  [unwired: 8 in]
                                }
                                }
                                n773 = case shown="True" w1060 {
                                tunnel: w1058 -> [w1100 w1112]
                                tunnel: [w1100 w1111] -> w1064
                                tunnel: w1059 -> [_ w1101]
                                frame False {
                                }
                                frame True {
                                n774 = disable-structure shown="Enabled" {
                                disable-tunnel: [w1122 w1123] -> w1102
                                disable-tunnel: w1101 -> [_ w1123]
                                frame Disabled {
                                n775 = local read item#-1() -> (w1122)
                                }
                                frame Enabled {
                                }
                                }
                                n776 = local read "pos_gps"() -> (w1106:dbl[])
                                n777 = call-poly <vilib>:"Array To Matrix.vi"("Real 1D Array"=w1112) -> ("Real Matrix (Column Vector)"=w1116:T14)
                                n778 = Array Subset(array=w1106, index=2, length=2) -> (w1107:dbl[])
                                n779 = Build Array (concatenate)(w1107, w1102) -> (w1103:dbl[])
                                n780 = global read "rio_Global.vi" "H"() -> (w1121:T14)
                                n781 = call-poly <vilib>:"Multiply.vi"("Real Matrix B"=w1116, "Real Matrix A"=w1121) -> ("A * B"=w1120:T14)
                                n782 = call-poly <vilib>:"Array To Matrix.vi"("Real 1D Array"=w1103) -> ("Real Matrix (Column Vector)"=w1119:T14)
                                n783 = call-poly <vilib>:"Subtract.vi"("Real Matrix B"=w1120, "Real Matrix A"=w1119) -> ("A - B"=w1117:T14)
                                n784 = global read "rio_Global.vi" "K"() -> (w1118:T14)
                                n785 = call-poly <vilib>:"Multiply.vi"("Real Matrix B"=w1117, "Real Matrix A"=w1118) -> ("A * B"=w1110:T14)
                                n786 = call-poly <vilib>:"Multiply.vi"("Real Matrix A"=w1110, "Real Scalar c"=0.25) -> ("c * A"=w1108:T14)
                                n787 = call-poly <vilib>:"Add.vi"("Real Matrix B"=w1116, "Real Matrix A"=w1108) -> ("A + B"=w1115:T14)
                                n788 = call-poly <vilib>:"Matrix To Array.vi"("Real Matrix"=w1115) -> ("Real 2D Array"=w1114:dbl[][])
                                n789 = Index Array(array=w1114, index (col)=0 ("disabled index (col)")) -> (element=w1111:dbl[])  [unwired: 1 in]
                                }
                                }
                                n790 = Replace Array Subset(array=w1064, new element=w1059, index=3) -> (w1062:dbl[])
                              }
                            }
                          }
                        }
                      }
                    }
                  }
                }
              }
            }
          }
          frame #2 {
            n791 = local read "h_gps"() -> (w1137:dbl)
            n792 = local read "dt"() -> (w1134:dbl)
            n793 = Index Array(array=w1148, index=3) -> (element=w1141:dbl)
            n794 = Array Subset(array=w1148, index=0, length=2) -> (→"pos":dbl[])
            n795 = Greater Than 0?(x=w1134) -> (x > 0?=w1133:bool)
            n796 = call "angleconv.vi"("rad"=w1141) -> ("deg"=→"Heading":dbl)  [unwired: 9 in, 1 out]
            n797 = Greater?(x=1.0, y=w1134) -> (0:w1136:bool)
            n798 = call "headingoperater.vi"("h1"=0.0, "h2"=w1137) -> ("h2+h1"=w1138:dbl)  [unwired: 8 in, 1 out]
            n799 = call "angleconv.vi"("rad"=w1138) -> ("deg"=→"H_GPS":dbl)  [unwired: 9 in, 1 out]
            n800 = Compound Arithmetic op=AND(w1136, w1133) -> (w1132:bool)
            n801 = case shown="True" w1132 {
              tunnel: w1148 -> [_ w1149]
              frame False {
              }
              frame True {
                n802 = flat-sequence {
                  tunnel: w1149 -> [w1173]
                  frame #0 {
                    n803 = Get Date/Time In Seconds() -> (seconds since 1Jan1904=w1164:timestamp)
                    n804 = To Double Precision Float(number=w1164) -> (double precision float=w1158:dbl)
                    n805 = global read "rio_Global.vi" "LCM_POS_T"() -> (w1172:T15)
                    n806 = local read "POS init"() -> (w1154:bool)
                    n807 = Unbundle By Name(w1172) -> ("hash"=w1169:i64)
                    n808 = local read "dt"() -> (w1153:dbl)
                    n809 = Multiply(x=w1158, y=1000000.0) -> (x*y=w1156:dbl)
                    n810 = Array To Cluster(array=w1173) -> (cluster=w1171:T16)
                    n811 = Select(t=0.0, s=w1154, f=w1153) -> (s? t:f=w1151:dbl)
                    n812 = call "hash.vi"("input"=w1169) -> ("output"=w1168:i64)  [unwired: 10 in]
                    n813 = To Quad Integer(1:w1156) -> (0:w1155:i64)
                    n814 = Unbundle(w1171) -> ("Real 2D Array[0]"=w1163:dbl, "Real 2D Array[1]"=w1162:dbl, "Real 2D Array[2]"=w1161:dbl, "Real 2D Array[3]"=w1160:dbl, "Real 2D Array[4]"=w1159:dbl)
                    n815 = Bundle(cluster=w1172, "hash"=w1168, "sys time"=w1155, "dt"=w1151, "x"=w1163, "y"=w1162, "speed"=w1161, "heading"=w1160, "yaw_rate"=w1159) -> (w1150:T15)
                    n816 = Flatten To String(anything=w1150, prepend array or string size? (T)=FALSE) -> (data string=w1166:string)  [unwired: 2 in, 2 out]
                    n817 = global read "rio_Global.vi" "LCM"() -> (w1165:T4)
                    n818 = call "LCM_send.vi"("DATA"=w1166, "ID"="POS_T", "LCM"=w1165) -> ()  [unwired: 7 in, 2 out]
                  }
                }
              }
            }
          }
        }
      }
    }
  }
